vi "Main.vi"() -> ()   [LabVIEW 2021]
uses:
  Program Files (x86)/National Instruments/LabVIEW 2021/examples/Design Patterns/Queued Message Handler/support/QMH Fundamentals - Message Cluster.ctl
  <vilib>/Utility/file.llb/Write Delimited Spreadsheet (string).vi
  <vilib>/Utility/xml.llb/Write to XML File(string).vi
  <vilib>/Utility/error.llb/Error Cluster From Error Code.vi
  <vilib>/Utility/xml.llb/Read From XML File(array).vi
  <vilib>/ErrorRing/Error Ring.xnode
panel:
  in  "bt_Manuel":bool caption="Manuel"
  out "boolEmergancyStop":bool caption="Acil Stop"
  out "bool_1":bool
  out "boolPollutionIndicator":bool caption="Kirlilik \nGöstergesi"
  out "boolMotorProtectionSwitch":bool caption="Motor\nKoruma Şalteri"
  in  "Bits":bool[](array[boolean])=[FALSE, FALSE, FALSE, FALSE, FALSE, FALSE, FALSE, FALSE, FALSE, FALSE, FALSE, FALSE, TRUE, FALSE, FALSE, FALSE, FALSE, TRUE, FALSE, FALSE, FALSE, FALSE, FALSE, TRUE, FALSE, FALSE, TRUE, TRUE, FALSE]
  in  "Languages":u16(ring)
  in  "Add Image":bool
  in  "bt_reportExcel":bool caption="Rapor"
  out "imagework":picture
  out "image testprm":picture
  in  "error in":errorcluster
  in  "bt_compare":bool caption="Karşılaştır"
  in  "bt_alarms":bool caption="Alarmlar"
  in  "bt_calibration":bool caption="Kalibrasyon"
  in  "bt_testStart":bool caption="Test Başlat"
  in  "bt_testStop":bool caption="Test Bitir"
  in  "bt_testPause":bool caption="Test Durdur"
  in  "bt_testCall":bool caption="Test Çağır"
  in  "bt_stopHydraulicSystem":bool caption="Sistem Durdur"
  in  "bt_startHydraulicSystem":bool caption="Sistem Başlat"
  in  "bt_exit":bool caption="ÇIKIŞ"
  in  "bt_home":bool caption="Home Button"
  in  "Pozisyon (Position)":dbl caption="Pozisyon" format="%#_g mm"
  in  "Kuvvet (Force)":dbl caption="Kuvvet" format="%#_6g N"
  out "Display Message":string="Test Edit" caption="DURUM BİLGİSİ"
  in  "General Tab":T1(tab)=enum."KalıpSeçimi"
  in  "General Pages Tab":T1(tab)=enum."KalıpSeçimi"
  in  "bt_continue":bool
  in  "Color Box":u32(colorbox)=12441574
  in  "Test Button General":enum32{"0", "1", "2"}(tab)=enum."1"
  in  "Test Pages Tab":enum32{"0", "1", "2", "3", "4", "5"}(tab)
  in  "KALIP BİLGİLERİ":T2={"Parça No"="Deneme2", "Seri No"="1", "Müşteri"="Mercedes-Benz", "Kalıp No"="6666", "Kuvvet Limiti [kN]"="1000", "Pres Tur"="15"} caption="t"
  in  "KONTROL PARAM":T3={"Kuvvet Limit"="Deneme2", "Grafik Limit"="1"}
  in  "String 2":string caption="Hız"
  in  "String":string caption="Pozisyon"
  in  "HAREKET PROFİLİ":T4 {"Bekleme Süresi" format="%#_g s"; "S3" format="%#_g mm/s"; "BDC" format="%#_g mm"; "S2" format="%#_g mm/s"; "P1" format="%#_g mm"; "S1" format="%#_g mm/s"; "TDC" format="%#_g mm"}
  in  "Image":i32(listbox) caption="Resim Seç"
  out "2D Picture":picture
  in  "bt_controlParameters":bool caption="Kontrol Parametreleri"
  in  "bt_moldInformation":bool caption="Kalıp Bilgileri"
  in  "bt_motionProfile":bool caption="Hareket Profili"
  in  "bt_recipeSave":bool caption="Kaydet"
  in  "bt_recipeSend":bool caption="Çalışmaya Gönder"
  in  "bt_recipeDelete":bool caption="Sil"
  in  "bt_graphLimited":bool caption="Grafik Sınırlayıcı"
  in  "bt_imageUpload":bool caption="Resim Yükle"
  in  "bt_newRecipe":bool caption="Yeni Kayıt"
  in  "Test Button Tab":enum32{"0", "1", "2", "3", "4", "5"}(tab)=enum."3"
  in  "bt_registrationPage":bool caption="Kayıt Sayfası"
  in  "bt_moldRecipeSearch":bool caption="Kalıp Ara"
  in  "searchRecipe":string="Deneme3"
  in  "moldSelection":i32(listbox)=2 caption="KALIP SEÇİMİ"
  in  "Mold Choice Tab":enum32{"0", "1"}(tab)=enum."1"
  out "pieceNo":string="Deneme2" caption="Parça No"
  out "serialNo":string="1" caption="Seri No"
  in  "bt_testEdit":bool caption="Testi Düzenle"
  out "Display Message 2":string="Test Edit" caption="Son Alarm"
  out "XY Graph":cluster{"X":dbl, "Y":dbl}[](graph)
  out "KALIP BİLGİLERİ-ÇALIŞMAs":T2={"Parça No"="Deneme2", "Seri No"="1", "Müşteri"="Mercedes-Benz", "Kalıp No"="6666", "Kuvvet Limiti [kN]"="1000", "Pres Tur"="15"} caption="KALIP BİLGİLERİ"
  in  "poliTestCheckbox":bool caption="Çoklu Test"
  in  "TEST PARAMETRELERİ":T5 caption="t" {"adet" format="%#_g mm"; "Min Kuvvet" format="%#_g kN"; "Max Kuvvet" format="%#_g kN"; "Min Pozisyon" format="%#_g mm"; "Max Pozisyon" format="%#_g mm"; "Kuvvet" format="%#_g kN"; "anlıkKuvvet" format="%#_g s"; "Hız" format="%#_g mm/s"; "tur" format="%#_g mm"}
  out "Comparexy":T6(graph)
  in  "deleteReferance":bool caption="Sil"
  out "Grafik Sayısı":string="2"
  in  "graphicReset":bool caption="Grafik Reset"
  in  "addReferance":bool caption="Grafik Ekle"
  in  "Alt Limit":string="30"
  in  "Referans Veriler":i32(listbox)=1
  in  "bt_AlarmsRemove":bool caption="REMOVE"
  in  "Alarms":i32(listbox) caption="ALARMLAR"
  in  "bt_CalibrationManuel":bool caption="MANUEL"
  in  "bt_CalibrationSave":bool caption="KAYDET"
  out "Cluster 3":T7 {"park_Position" format="%#_g s"; "decomp_CycleTime" format="%#_g s"; "YEDEK" format="%#_g s"; "YEDEK" format="%#_g s"; "YEDEK" format="%#_g h"; "decomp_Cycle" format="%#_g s"; "p6_Druck" format="%#_g s"; "auffahren_Druck" format="%#_g h"; "press_Druck" format="%#_g s"; "langsam_Druck" format="%#_g mm"; "Schnellabdruck" format="%#_g bar"; "low_Temp" format="%#_g kN"; "fan_StopTemp" format="%#_g bar"; "fan_StartTemp" format="%#_g mm"}
  in  "Cluster 2":T8
  out "Cluster":T9 {"YEDEK" format="%#_g s"; "YEDEK" format="%#_g bar"; "YEDEK" format="%#_g kN"; "Wait" format="%#_g s"; "working_Time" format="%#_g h"; "Time" format="%#_g s"; "min_PosD" format="%#_g mm"; "pressure_Bd" format="%#_g bar"; "Kraftd" format="%#_g kN"; "pressure_Name" format="%#_g bar"; "Position" format="%#_g mm"}
  out "Table Control 2":string[][](table) caption="Table Control"
  out "Table Control":string[][](table)
  # "NOTLAR\n1- Otomatik sayfası eklenecek (climatic testteki gibi)\n2- Ayarlar sayfasındaki fan start clusteri gizle ve Pega climaticteki kalibrasyon sayfasındaki\ngibi input ve output boolean değişkenleri ekle\n3- Grafik sınırlayıcıyı fıratın anlattığı ve attığı videolardaki gibi yap\n4-"
  # "V 0.0.0.1"
  # "MSP-120-S-HCD\n120kN Servo Press"
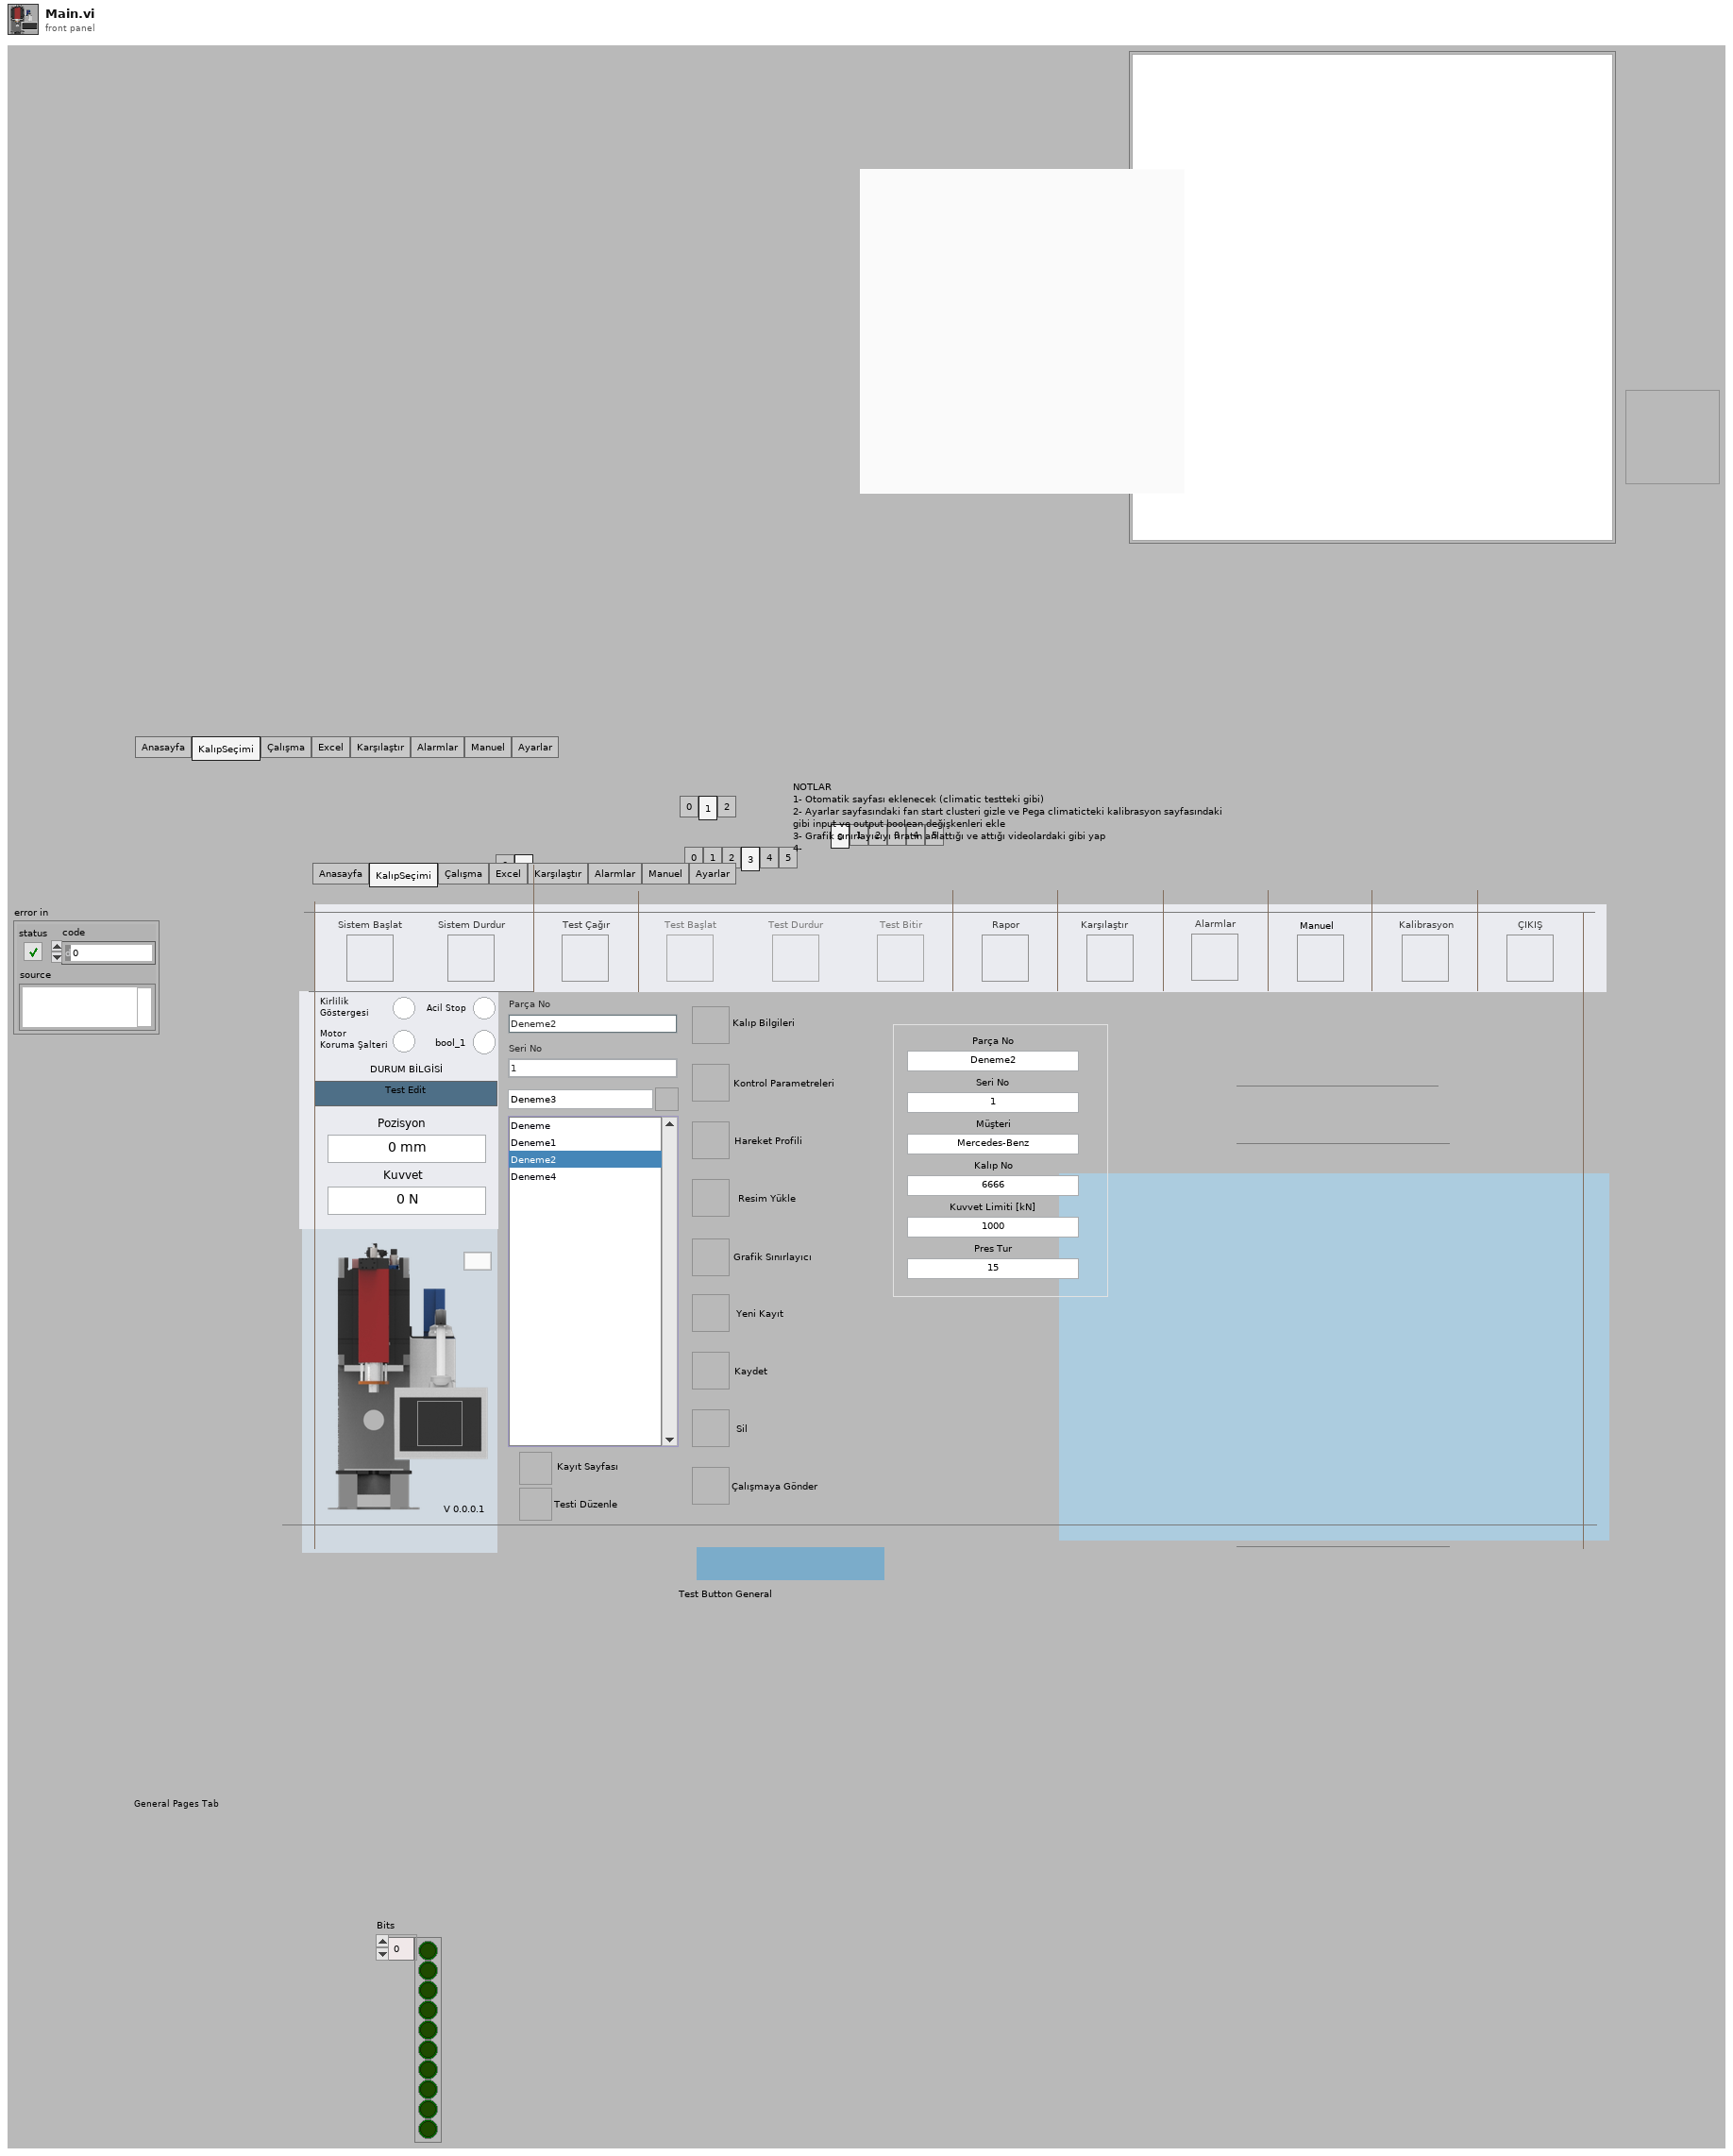
[diagram p1: front panel]
types:
  T1 = enum32{"Anasayfa", "KalıpSeçimi", "Çalışma", "Excel", "Karşılaştır", "Alarmlar", "Manuel", "Ayarlar"}
  T2 = cluster{"Parça No":string, "Seri No":string, "Müşteri":string, "Kalıp No":string, "Kuvvet Limiti [kN]":string, "Pres Tur":string}
  T3 = cluster{"Kuvvet Limit":string, "Grafik Limit":string}
  T4 = cluster{"TDC":dbl, "S1":dbl, "P1":dbl, "S2":dbl, "BDC":dbl, "S3":dbl, "Bekleme Süresi":dbl}
  T5 = cluster{"tur":dbl, "Hız":dbl, "anlıkKuvvet":dbl, "Kuvvet":dbl, "Max Pozisyon":dbl, "Min Pozisyon":dbl, "Max Kuvvet":dbl, "Min Kuvvet":dbl, "adet":dbl}
  T6 = cluster{"Item Names":dbl[], "Item Names":dbl[]}[]
  T7 = cluster{"fan_StartTemp":dbl, "fan_StopTemp":dbl, "over_Temp":dbl, "low_Temp":dbl, "Schnellabdruck":dbl, "langsam_Druck":dbl, "press_Druck":dbl, "auffahren_Druck":dbl, "p5_Druck":dbl, "p6_Druck":dbl, "decomp_Cycle":dbl, "YEDEK":dbl, "YEDEK":dbl, "YEDEK":dbl, "YEDEK":dbl, "decomp_CycleTime":dbl, "park_Position":dbl}
  T8 = cluster{"jog_Press":bool, "Fgrenze":bool, "start_HoldTime":bool, "move_DoneForce":bool, "hold_TimeDone":bool, "start_Decomp":bool, "decompJog":bool, "Startup":bool, "Motion":bool, "Lamp":bool, "reset_Axis":bool, "YEDEK":bool, "YEDEK":bool, "YEDEK":bool}
  T9 = cluster{"Position":dbl, "pressure_Name":dbl, "total_Parts":dbl, "Kraftd":dbl, "pressure_Bd":dbl, "min_PosD":dbl, "Time":dbl, "working_Time":dbl, "max_Force":dbl, "Wait":dbl, "YEDEK":dbl, "YEDEK":dbl, "YEDEK":dbl, "YEDEK":dbl}
  T10 = typedef "QMH Fundamentals - Message Cluster.ctl" = cluster{"Message":string, "Message Data":variant}
  T11 = enum16{"open", "replace", "create", "open or create", "replace or create", "replace or create with confirmation"}
  T12 = cluster{"Parça No":string, "Seri No":string, "Müşteri":string, "Kalıp No":string, "Kuvvet Limiti [kN]":string, "Kuvvet Limiti [kN] 2":string}
  T13 = cluster{"KALIP BİLGİLERİ 2":cluster{"Parça No":string, "Seri No":string, "Müşteri":string, "Kalıp No":string, "Kuvvet Limiti [kN]":string, "Kuvvet Limiti [kN] 2":string}, "Parça No":string, "Seri No":string, "KALIP BİLGİLERİ":cluster{"Kuvvet Limiti [kN]":string, "Kuvvet Limiti [kN] 2":string}, "HAREKET PROFİLİ":cluster{"TDC":dbl, "S1":dbl, "P1":dbl, "S2":dbl, "BDC":dbl, "S3":dbl, "Bekleme Süresi":dbl}, "new picture":picture, "picture index":dbl}
  T14 = cluster{"Kuvvet Limiti [kN]":string, "Kuvvet Limiti [kN] 2":string}
  T15 = enum8{"Enabled", "Disabled", "Disabled and Grayed Out"}
  T16 = typedef "imagedata.ctl" = cluster{"image type":i32, "image depth":i32, "image":u8[], "mask":u8[], "colors":u32[], "Rectangle":cluster{"left":i16, "top":i16, "right":i16, "bottom":i16}}
  T17 = cluster{"Parça No":string, "Seri No":string, "Müşteri":string, "Kalıp No":string, "Kuvvet Limiti [kN]":string}
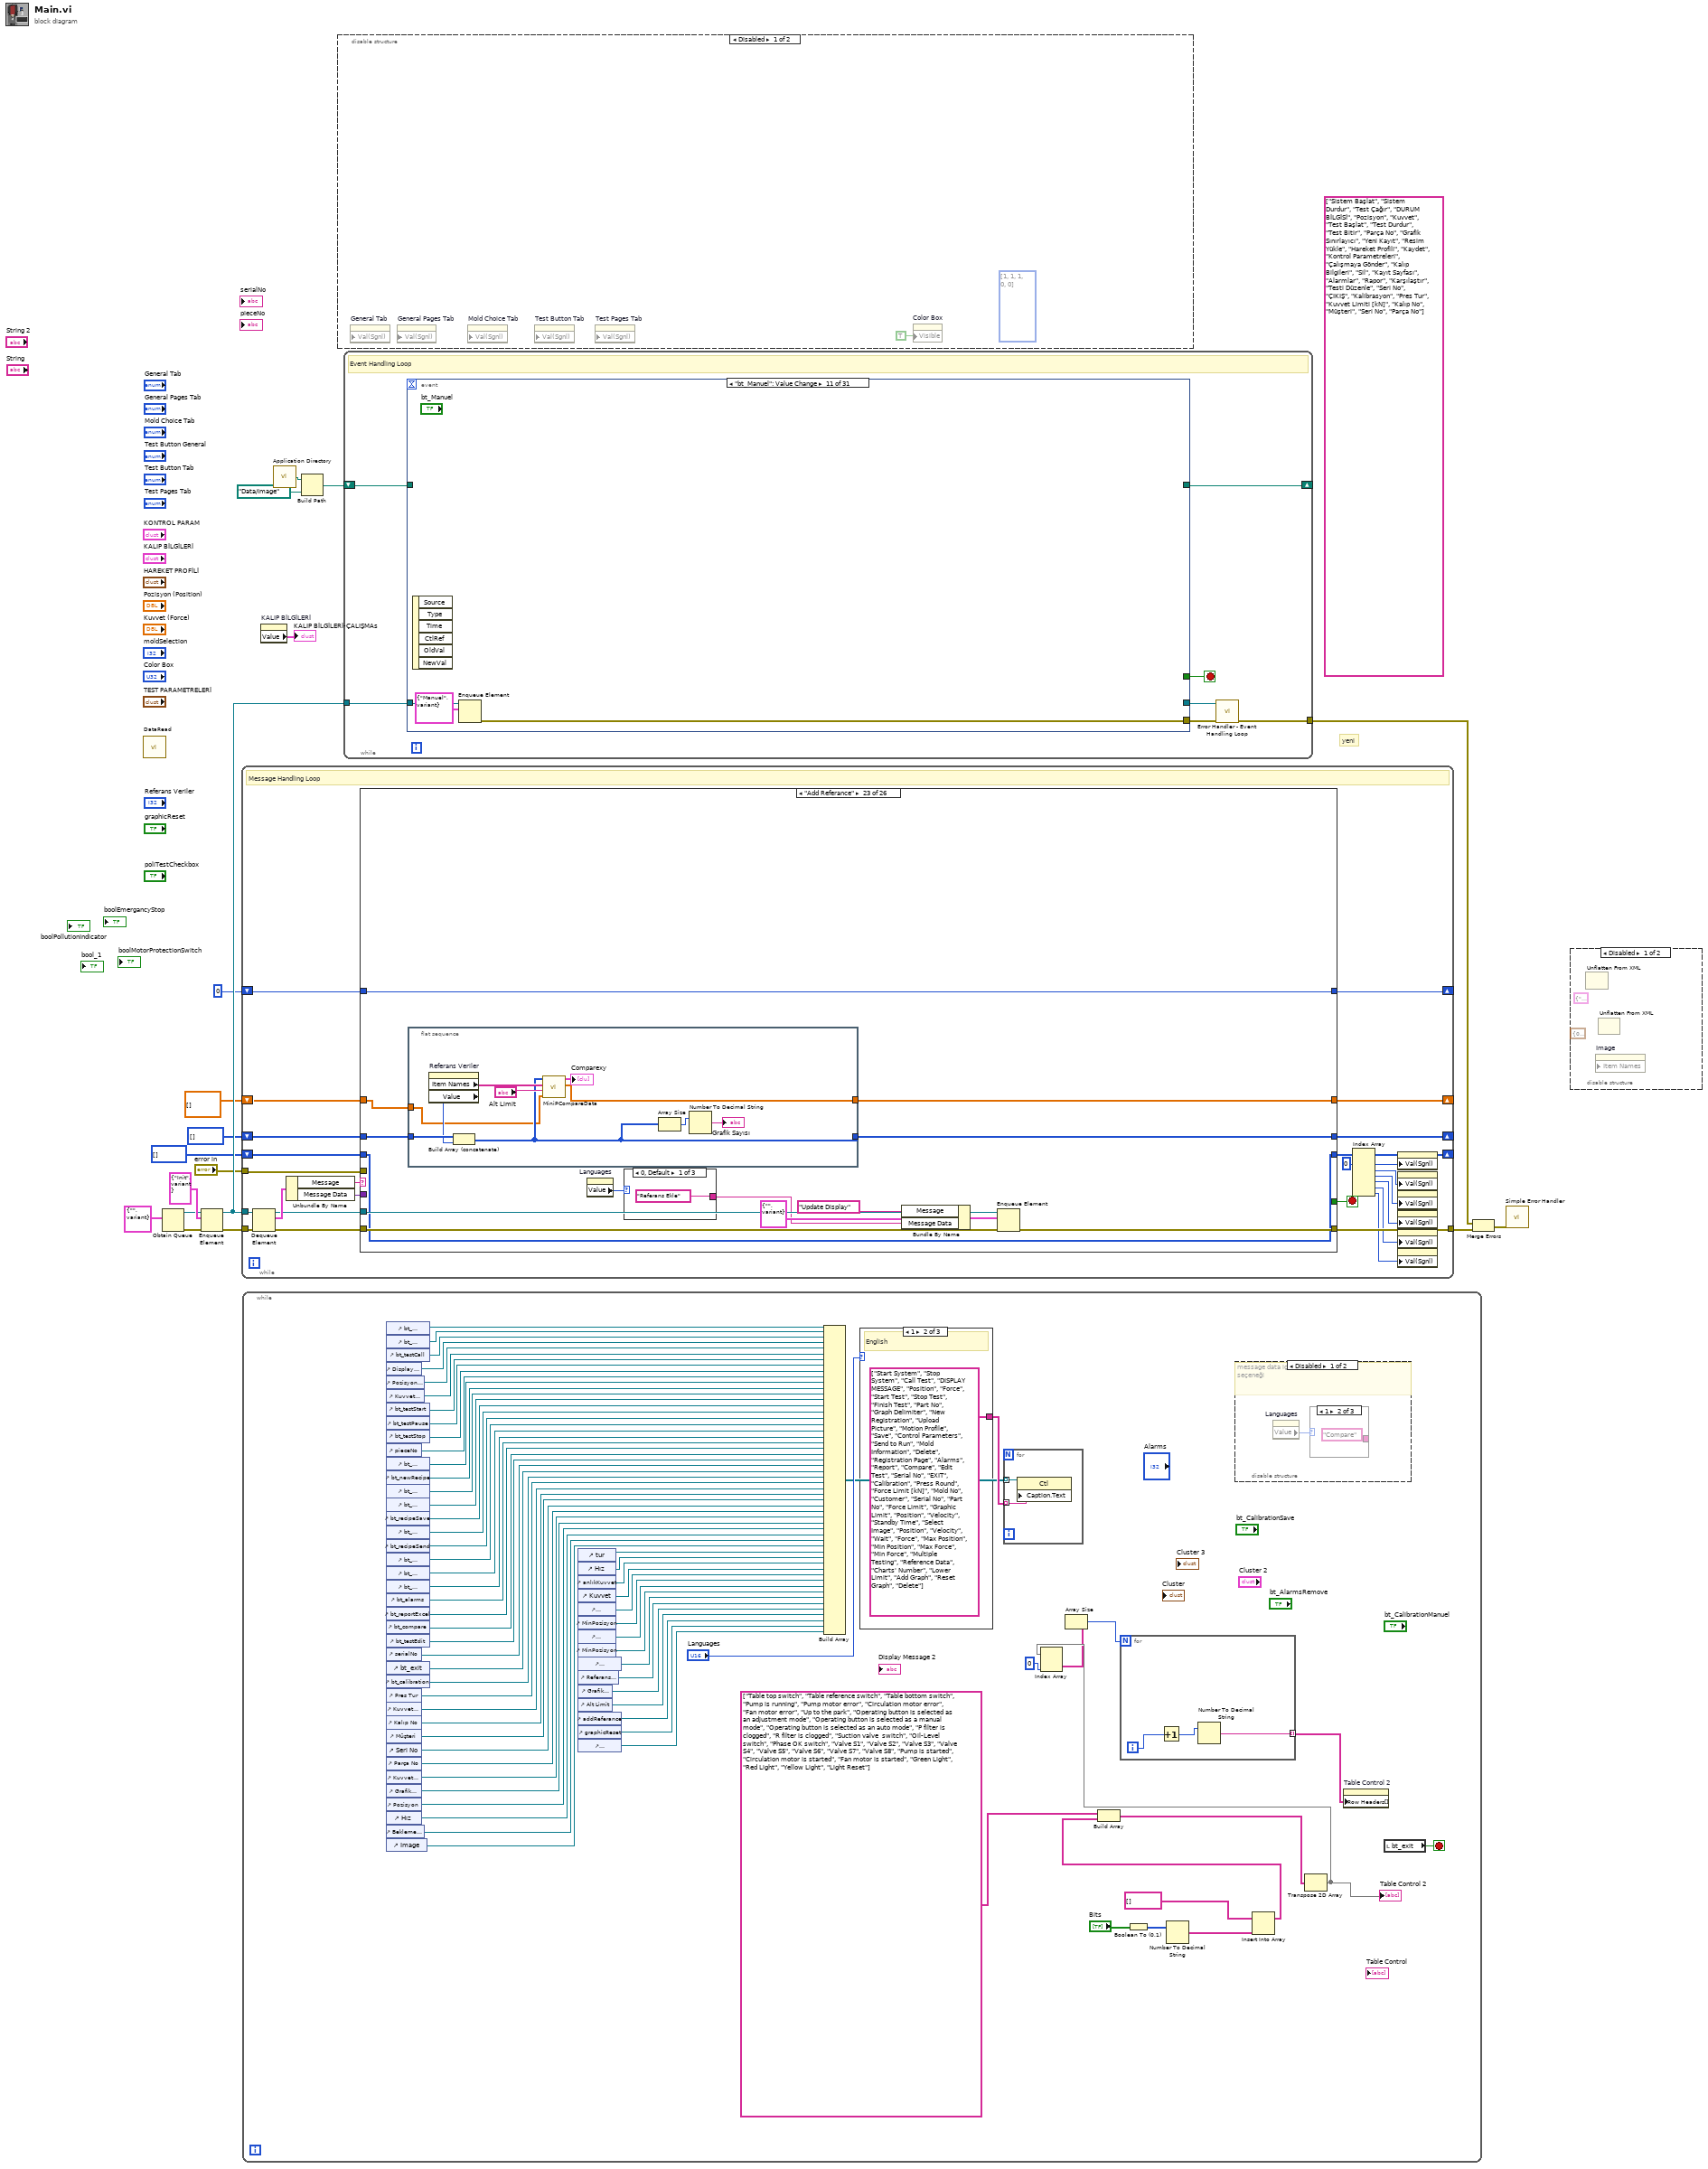
[diagram p0: block diagram]
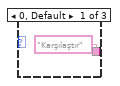
[diagram p2: hidden frame]
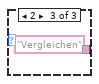
[diagram p3: hidden frame]
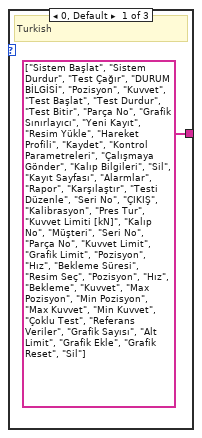
[diagram p5: hidden frame]
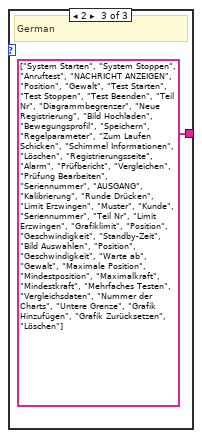
[diagram p6: hidden frame]
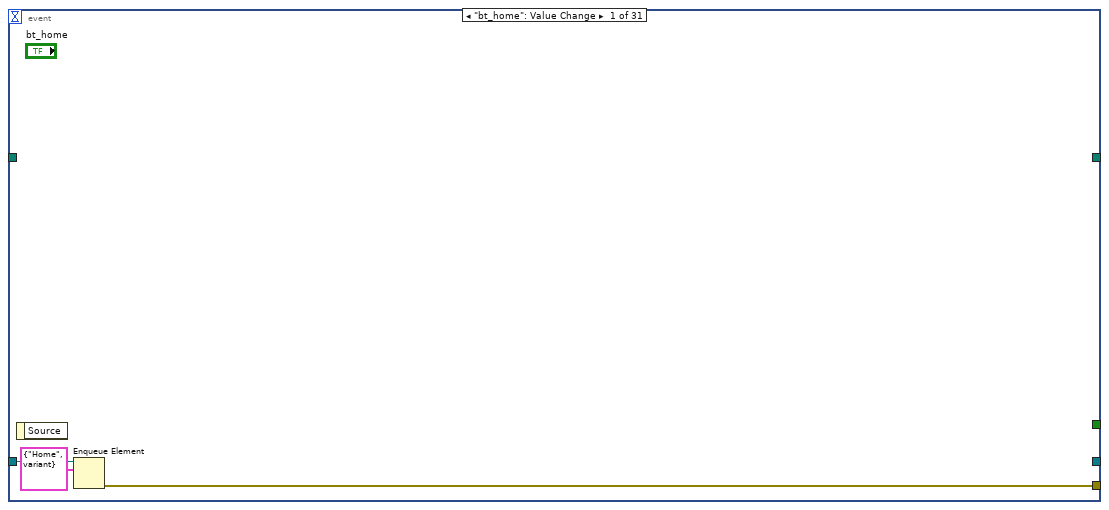
[diagram p9: hidden frame]
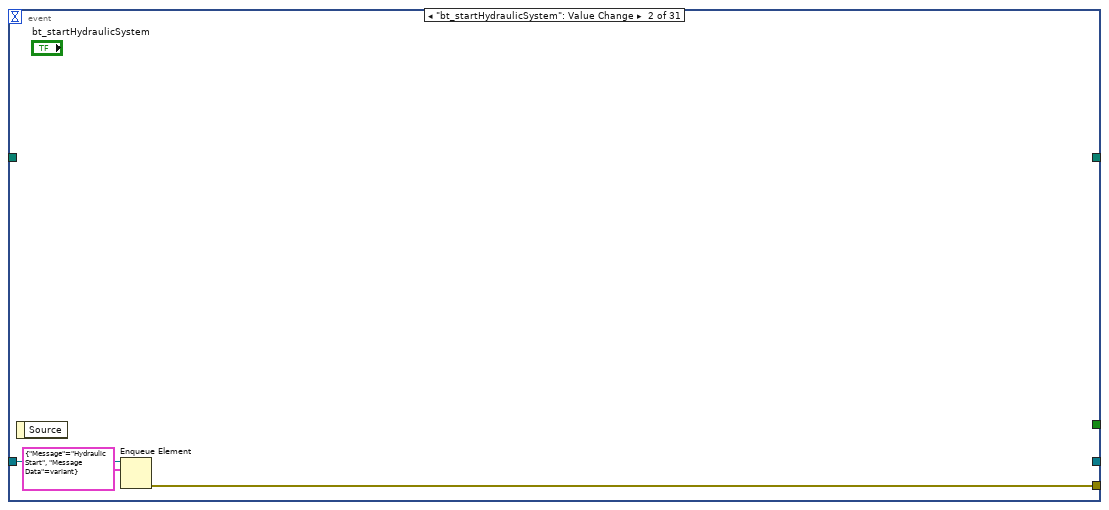
[diagram p10: hidden frame]
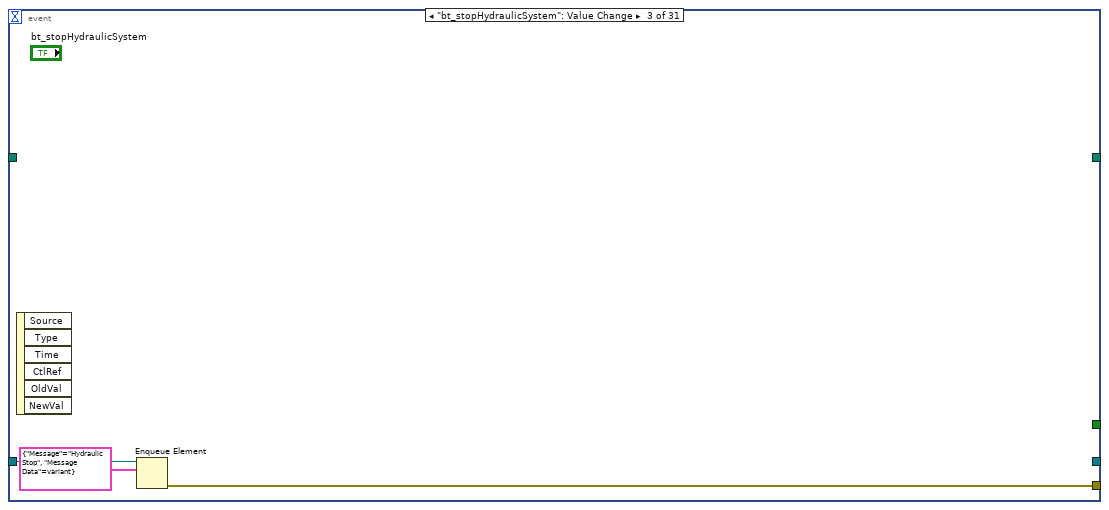
[diagram p11: hidden frame]
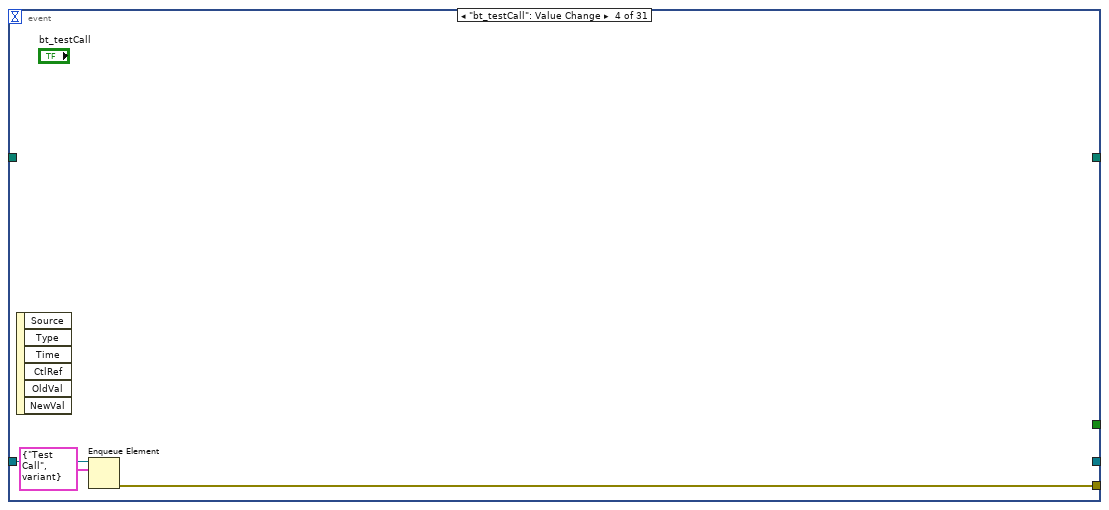
[diagram p12: hidden frame]
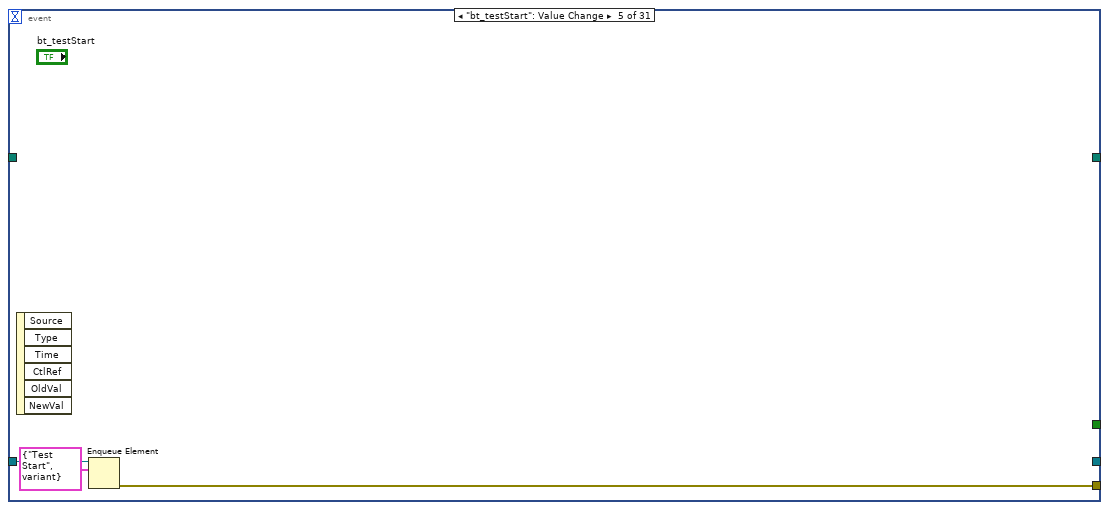
[diagram p13: hidden frame]
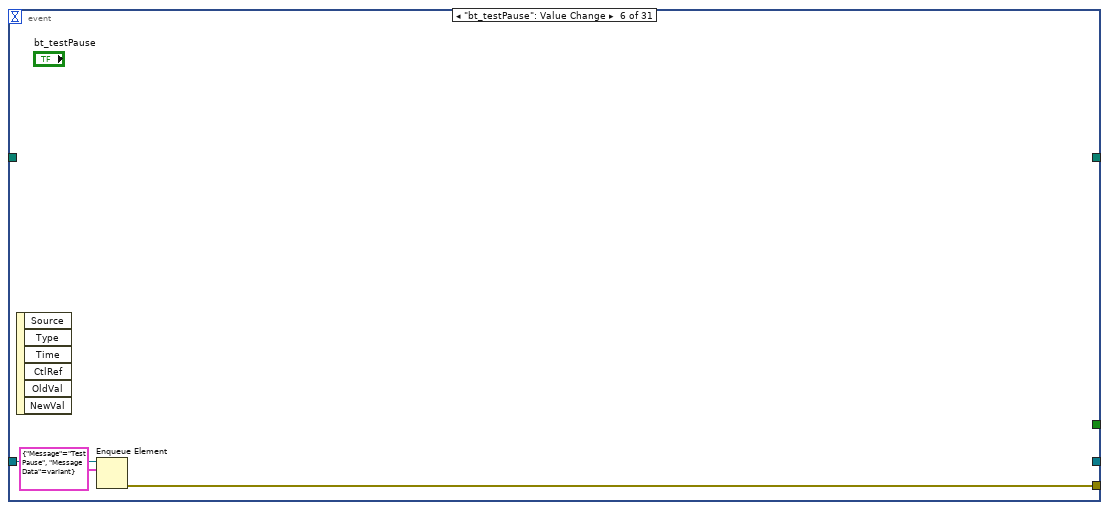
[diagram p14: hidden frame]
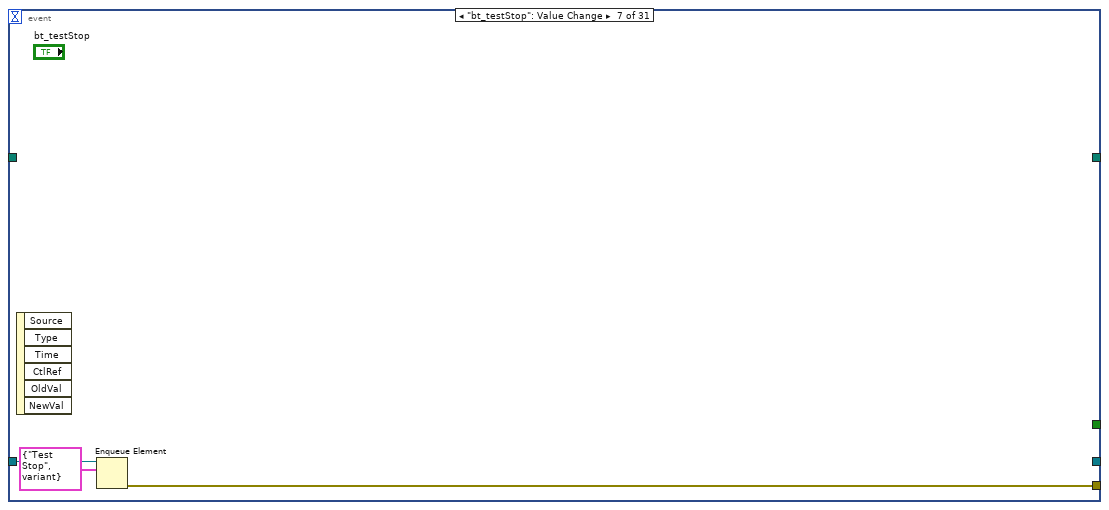
[diagram p15: hidden frame]
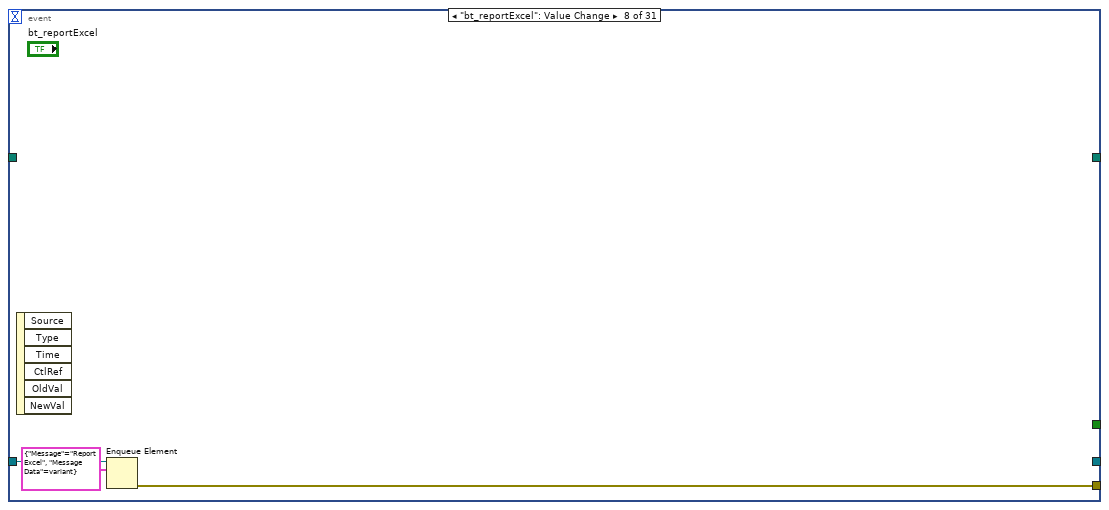
[diagram p16: hidden frame]
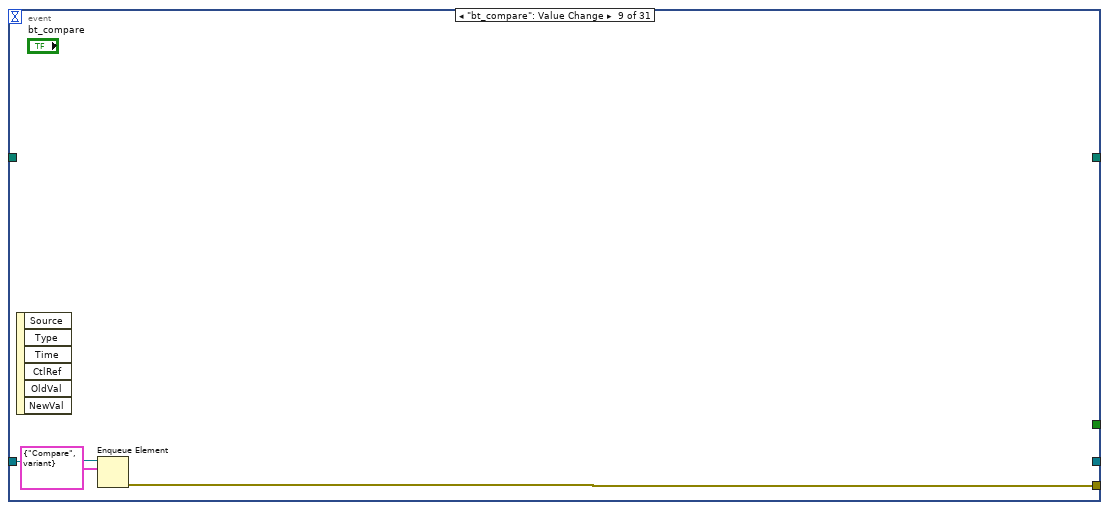
[diagram p17: hidden frame]
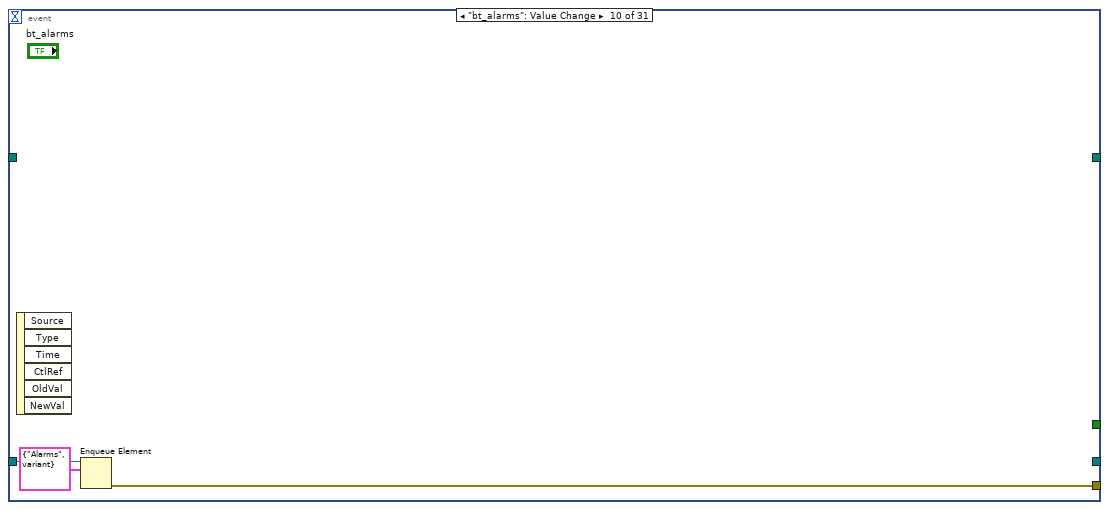
[diagram p18: hidden frame]
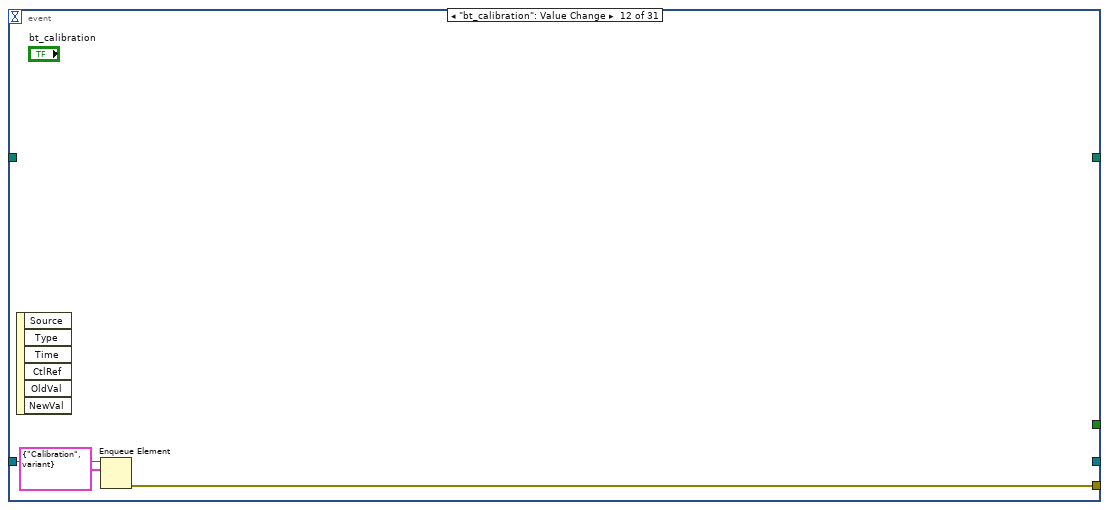
[diagram p19: hidden frame]
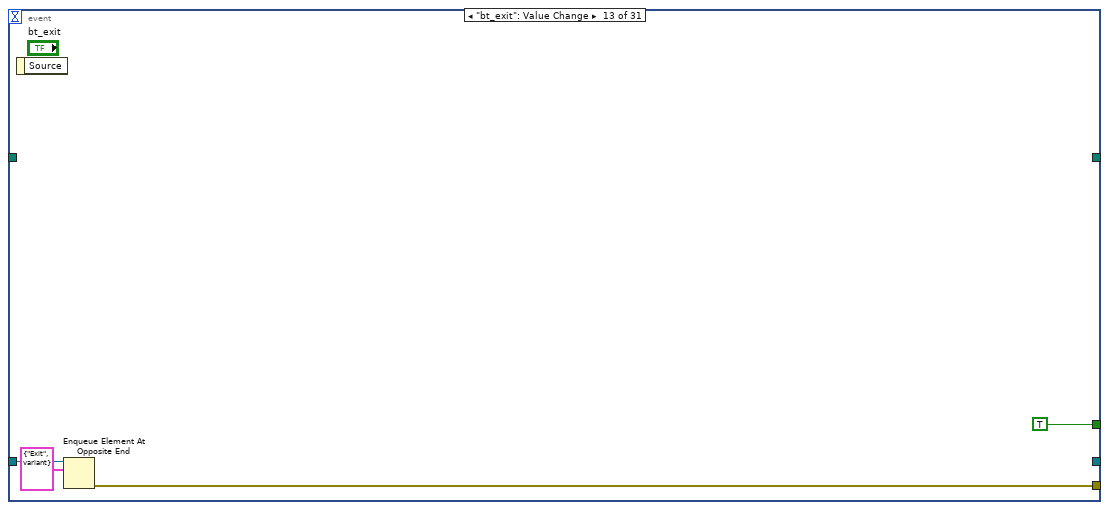
[diagram p20: hidden frame]
diagram:
  (unwired) string[] ["Sistem Başlat", "Sistem Durdur", "Test Çağır", "DURUM BİLGİSİ", "Pozisyon", "Kuvvet", "Test Başlat", "Test Durdur", "Test Bitir", "Parça No", "Grafik Sınırlayıcı", "Yeni Kayıt", "Resim Yükle", "Hareket Profili", "Kaydet", "Kontrol Parametreleri", "Çalışmaya Gönder", "Kalıp Bilgileri", "Sil", "Kayıt Sayfası", "Alarmlar", "Rapor", "Karşılaştır", "Testi Düzenle", "Seri No", "ÇIKIŞ", "Kalibrasyon", "Pres Tur", "Kuvvet Limiti [kN]", "Kalıp No", "Müşteri", "Seri No", "Parça No"] ("appended array")
  # "yeni"
  n1 = call "DataRead.vi"() -> ()  [unwired: 12 in]
  n2 = Obtain Queue(element data type=T10 {"Message"="", "Message Data"=variant} ("Message Cluster")) -> (queue out=w11:refnum<queue>, error out=w10:errorcluster)  [unwired: 4 in, 1 out]
  n3 = Enqueue Element(queue=w11, element=T10 {"Message"="Init", "Message Data"=variant}, error in (no error)=w10) -> (queue out=w15:refnum<queue>, error out=w16:errorcluster)  [unwired: 1 in, 1 out]
  n4 = while {
    tunnel: w15 -> [w40]
    tunnel: w16 -> [w41]
    tunnel: [w42] -> w18
    tunnel: "error in" -> [w34]
    shift-right: [w31] -> _
    shift-left: i32[] [] -> [w30]
    shift-right: [w23] -> _
    shift-left: i32[] [] -> [w24]
    shift-right: [w22] -> _
    shift-left: dbl[][] [] ("output array 3") -> [w19]
    shift-right: [w20] -> _
    shift-left: 0 -> [w21]
    stop <- w43 stop-if-true
    # "Message Handling Loop"
    n5 = Dequeue Element(queue=w40, error in (no error)=w41) -> (queue out=w38:refnum<queue>, element=w39:T10, error out=w37:errorcluster)  [unwired: 1 in, 1 out]
    n6 = Unbundle By Name(w39) -> ("Message"=w36:string, "Message Data"=w35:variant)
    n7 = case "Message Cases" shown="\"Add Referance\"" w36 {
      selector: w36 -> [_ _ _ _ _ _ _ _ _ _ _ _ _ _ _ _ _ _ _ _ _ _ _ _ _ w671]
      tunnel: w38 -> [_ w63 w78 w93 w113 w128 w143 w158 w214 w252 w290 w306 w321 w334 w349 w366 w418 w433 w456 w505 w558 w601 w618 w645 _ _]
      tunnel: w37 -> [w51 w61 w76 w91 w111 w126 w141 w156 w212 w250 w288 w304 w319 w331 w347 w364 w416 w431 w455 w504 w556 w599 w616 w643 w664 w670]
      tunnel: [w51 w62 w77 w92 w112 w127 w142 w157 w213 w251 w289 w305 w320 w332 w348 w365 w417 w432 w442 w492 w557 w600 w617 w644 w662 w670] -> w42
      tunnel: [_ _ _ _ _ _ _ _ _ _ _ _ _ TRUE _ _ _ _ _ _ _ _ _ _ _ _] -> w43
      tunnel: w35 -> [_ _ _ _ _ _ _ _ _ _ _ _ _ _ _ _ _ _ _ _ _ _ _ _ w663 _]
      tunnel: w34 -> [_ _ _ _ _ _ _ _ w163 _ w279 w295 _ _ _ _ _ _ w451 _ _ _ _ _ _ _]
      tunnel: [i32[] [0, 0, 0, 0, 0] i32[] [0, 0, 0, 0, 0] w72 w87 w103 w122 w137 w152 w208 i32[] [4, 4, 0, 1, 0] i32[] [5, 5, 0, 1, 0] i32[] [6, 6, 0, 1, 0] i32[] [7, 7, 0, 1, 0] w330 i32[] [1, 1, 0, 5, 5] w357 w407 i32[] [1, 1, 1, 1, 0, 0] w446 w483 w552 i32[] [2, 2, 1, 1, 0] w612 w639 w660 w668] -> w31
      tunnel: w30 -> [_ _ w72 w87 w102 w122 w137 w152 w208 _ _ _ _ w330 _ w358 w412 _ w445 w488 w552 _ w612 w639 w660 w668]
      tunnel: w24 -> [w48 w56 w71 w86 w101 w121 w136 w151 w207 w245 w283 w299 w314 w329 w342 w359 w406 w426 w441 w482 w551 w594 w611 w638 w659 w667]
      tunnel: [w48 w56 w71 w86 w101 w121 w136 w151 w207 w245 w283 w299 w314 w329 w342 w359 w406 w426 w441 w482 w551 w594 w610 w636 w659 w667] -> w23
      tunnel: w19 -> [w45 w55 w70 w85 w100 w120 w135 w150 w175 w244 w282 w298 w313 w328 w341 w356 w405 w425 w440 w481 w550 w593 w605 w635 w657 w666]
      tunnel: [w45 w55 w70 w85 w100 w120 w135 w150 w175 w244 w282 w298 w313 w328 w341 w356 w405 w425 w440 w481 w550 w593 w606 w634 w657 w666] -> w22
      tunnel: w21 -> [w44 w54 w69 w84 w99 w119 w134 w149 w169 w243 w281 w297 w312 w327 w340 w355 w404 w424 w439 w480 w549 w592 w609 w637 w656 w665]
      tunnel: [w44 w54 w69 w84 w99 w119 w134 w149 w165 w243 w281 w297 w312 w327 w340 w355 w404 w424 w439 w480 w549 w592 w609 w637 w656 w665] -> w20
      frame "Init" {
        # "Initialize - Perform any initialization code for your application here. In this example, the only initialization required is setting the Display Message indicator value to an empty string."
        n8 = property on="moldSelection" class="LstBox (strict)"("Value"=nan) -> ()  [unwired: 2 in, 2 out]
        n9 = property on="Test Button General" class="TabCtl (strict)"("Val(Sgnl)"=enum32{"0", "1", "2"}."0" ("Value (Signaling)")) -> ()  [unwired: 2 in, 2 out]
        n10 = local write "Display Message"("") -> ()
      }
      frame "Home" {
        # "Action 1 - Send an \"Update Display\" message indicating which button was pressed. Note that a string is sent as the Message Data along with the \"Update Display\" message."
        n11 = property on="Languages" class="Ring (strict)"() -> ("Value"=w53:u16)  [unwired: 2 in, 2 out]
        n12 = case shown="0, Default" w53 {
          tunnel: ["Ev" ("L10n_Action 2 Pressed") "Home" ("L10n_Action 2 Pressed") "Heim" ("L10n_Action 2 Pressed")] -> w52
          frame 0, Default {
          }
          frame 1 {
          }
          frame 2 {
          }
        }
        n13 = Bundle By Name(cluster=T10 {"Message"="", "Message Data"=variant} ("Message Cluster"), "Message"="Update Display", "Message Data"=w52) -> (w58:T10)
        n14 = Enqueue Element(queue=w63, element=w58, error in (no error)=w61) -> (error out=w62:errorcluster)  [unwired: 1 in, 2 out]
      }
      frame "Hydraulic Start" {
        # "Action 1 - Send an \"Update Display\" message indicating which button was pressed. Note that a string is sent as the Message Data along with the \"Update Display\" message."
        n15 = property on="Languages" class="Ring (strict)"() -> ("Value"=w68:u16)  [unwired: 2 in, 2 out]
        n16 = case shown="2" w68 {
          tunnel: ["Hidrolik Başlat" ("L10n_Action 2 Pressed") "Hydraulic Start" ("L10n_Action 2 Pressed") "Hydraulik Starten" ("L10n_Action 2 Pressed")] -> w67
          frame 0, Default {
          }
          frame 1 {
          }
          frame 2 {
          }
        }
        n17 = Bundle By Name(cluster=T10 {"Message"="", "Message Data"=variant} ("Message Cluster"), "Message"="Update Display", "Message Data"=w67) -> (w73:T10)
        n18 = Enqueue Element(queue=w78, element=w73, error in (no error)=w76) -> (error out=w77:errorcluster)  [unwired: 1 in, 2 out]
      }
      frame "Hydraulic Stop" {
        # "Action 2 - Send an \"Update Display\" message indicating which button was pressed. Note that a string is sent as the Message Data along with the \"Update Display\" message."
        n19 = property on="Languages" class="Ring (strict)"() -> ("Value"=w83:u16)  [unwired: 2 in, 2 out]
        n20 = case shown="2" w83 {
          tunnel: ["Hidrolik Durdur" ("L10n_Action 2 Pressed") "Hydraulic Stop" ("L10n_Action 2 Pressed") "Hydraulik Stoppen" ("L10n_Action 2 Pressed")] -> w82
          frame 0, Default {
          }
          frame 1 {
          }
          frame 2 {
          }
        }
        n21 = Bundle By Name(cluster=T10 {"Message"="", "Message Data"=variant} ("Message Cluster"), "Message"="Update Display", "Message Data"=w82) -> (w88:T10)
        n22 = Enqueue Element(queue=w93, element=w88, error in (no error)=w91) -> (error out=w92:errorcluster)  [unwired: 1 in, 2 out]
      }
      frame "Test Call" {
        # "Action 2 - Send an \"Update Display\" message indicating which button was pressed. Note that a string is sent as the Message Data along with the \"Update Display\" message."
        n23 = property on="Languages" class="Ring (strict)"() -> ("Value"=w98:u16)  [unwired: 2 in, 2 out]
        n24 = case shown="2" w98 {
          tunnel: ["Test Çağır" ("L10n_Action 2 Pressed") "Call Test" ("L10n_Action 2 Pressed") "Anruftest" ("L10n_Action 2 Pressed")] -> w97
          frame 0, Default {
          }
          frame 1 {
          }
          frame 2 {
          }
        }
        n25 = Replace Array Subset(array=w102, new element #1=1 ("new element/subarray"), index #1=0 ("index"), new element #2=1 ("new element/subarray"), index #2=1 ("index")) -> (w103:i32[])
        n26 = Bundle By Name(cluster=T10 {"Message"="", "Message Data"=variant} ("Message Cluster"), "Message"="Update Display", "Message Data"=w97) -> (w108:T10)
        n27 = Enqueue Element(queue=w113, element=w108, error in (no error)=w111) -> (error out=w112:errorcluster)  [unwired: 1 in, 2 out]
      }
      frame "Test Start" {
        # "Action 2 - Send an \"Update Display\" message indicating which button was pressed. Note that a string is sent as the Message Data along with the \"Update Display\" message."
        n28 = property on="Languages" class="Ring (strict)"() -> ("Value"=w118:u16)  [unwired: 2 in, 2 out]
        n29 = case shown="2" w118 {
          tunnel: ["Test Başlat" ("L10n_Action 2 Pressed") "Test Start" ("L10n_Action 2 Pressed") "Test Starten" ("L10n_Action 2 Pressed")] -> w117
          frame 0, Default {
          }
          frame 1 {
          }
          frame 2 {
          }
        }
        n30 = Bundle By Name(cluster=T10 {"Message"="", "Message Data"=variant} ("Message Cluster"), "Message"="Update Display", "Message Data"=w117) -> (w123:T10)
        n31 = Enqueue Element(queue=w128, element=w123, error in (no error)=w126) -> (error out=w127:errorcluster)  [unwired: 1 in, 2 out]
      }
      frame "Test Pause" {
        # "Action 2 - Send an \"Update Display\" message indicating which button was pressed. Note that a string is sent as the Message Data along with the \"Update Display\" message."
        n32 = property on="Languages" class="Ring (strict)"() -> ("Value"=w133:u16)  [unwired: 2 in, 2 out]
        n33 = case shown="0, Default" w133 {
          tunnel: ["Test Durdur" ("L10n_Action 2 Pressed") "Test Pause" ("L10n_Action 2 Pressed") "Test Stoppen" ("L10n_Action 2 Pressed")] -> w132
          frame 0, Default {
          }
          frame 1 {
          }
          frame 2 {
          }
        }
        n34 = Bundle By Name(cluster=T10 {"Message"="", "Message Data"=variant} ("Message Cluster"), "Message"="Update Display", "Message Data"=w132) -> (w138:T10)
        n35 = Enqueue Element(queue=w143, element=w138, error in (no error)=w141) -> (error out=w142:errorcluster)  [unwired: 1 in, 2 out]
      }
      frame "Test Stop" {
        # "Action 2 - Send an \"Update Display\" message indicating which button was pressed. Note that a string is sent as the Message Data along with the \"Update Display\" message."
        n36 = property on="Languages" class="Ring (strict)"() -> ("Value"=w148:u16)  [unwired: 2 in, 2 out]
        n37 = case shown="2" w148 {
          tunnel: ["Test Bitir" ("L10n_Action 2 Pressed") "Test Beenden" ("L10n_Action 2 Pressed") "Finish Test" ("L10n_Action 2 Pressed")] -> w147
          frame 0, Default {
          }
          frame 1 {
          }
          frame 2 {
          }
        }
        n38 = Bundle By Name(cluster=T10 {"Message"="", "Message Data"=variant} ("Message Cluster"), "Message"="Update Display", "Message Data"=w147) -> (w153:T10)
        n39 = Enqueue Element(queue=w158, element=w153, error in (no error)=w156) -> (error out=w157:errorcluster)  [unwired: 1 in, 2 out]
      }
      frame "Report Excel" {
        # "Action 2 - Send an \"Update Display\" message indicating which button was pressed. Note that a string is sent as the Message Data along with the \"Update Display\" message."
        n40 = property on="Languages" class="Ring (strict)"(error in=w163) -> ("Value"=w164:u16)  [unwired: 1 in, 2 out]
        n41 = Increment(x=w169) -> (x+1=w165:i32)
        n42 = case shown="2" w164 {
          tunnel: ["Excele Raporla" ("L10n_Action 2 Pressed") "Report Excel" ("L10n_Action 2 Pressed") "Prüfbericht Excel" ("L10n_Action 2 Pressed")] -> w162
          frame 0, Default {
          }
          frame 1 {
          }
          frame 2 {
          }
        }
        n43 = Number To Decimal String(number=w165) -> (decimal integer string=w167:string)  [unwired: 1 in]
        n44 = Bundle By Name(cluster=T10 {"Message"="", "Message Data"=variant} ("Message Cluster"), "Message"="Update Display", "Message Data"=w162) -> (w209:T10)
        n45 = disable-structure shown="Disabled" {
          frame Disabled {
            (unwired) dbl[][] [[244.257944, 45.058472], [244.257944, 45.058472], [244.507425, 58.662598], [244.757021, 77.658325], [245.006311, 94.001465], [245.25667, 114.316162], [245.507105, 131.029785], [245.757044, 151.04895], [246.006906, 167.49231], [246.256769, 187.022217], [246.507318, 202.838623], [246.757372, 221.95752], [247.006471, 237.069092], [247.257021, 255.672485], [247.507189, 270.313477], [247.757128, 288.54126], [248.007219, 302.773437], [248.2567, 320.695068], [248.507364, 334.658569], [248.757532, 352.358887], [249.00667, 366.036377], [249.257448, 383.486328], [249.507044, 397.035278], [249.757326, 414.338745], [250.007417, 427.50415], [250.256822, 444.507324], [250.507562, 457.680054], [250.757463, 474.576172], [251.00683, 487.561768], [251.257379, 504.411011], [251.507013, 517.157349], [251.757181, 533.88916], [252.007463, 546.530029], [252.256868, 563.121338], [252.507532, 575.629883], [252.757318, 592.188599], [253.006723, 604.656616], [253.257387, 621.057129], [253.507326, 633.444458], [253.757112, 649.878906], [254.007547, 662.192505], [254.25699, 678.359985], [254.507463, 690.679443], [254.757402, 706.931396], [255.006807, 719.049927], [255.257395, 735.057617], [255.507257, 747.286377], [255.757273, 763.268311], [256.007631, 775.393555], [256.256883, 791.341064], [256.507433, 803.436523], [256.757486, 819.349731], [257.006853, 831.404297], [257.257326, 847.233398], [257.507189, 859.23291], [257.75728, 875.164185], [258.007601, 887.022461], [258.256853, 902.898071], [258.507364, 914.703979], [258.757532, 930.603638], [259.006784, 942.289917], [259.257372, 958.166626], [259.507234, 969.790161], [259.757402, 985.563843], [260.007379, 997.39856], [260.256746, 1013.030029], [260.507334, 1024.908203], [260.757311, 1040.422485], [261.006944, 1052.170166], [261.257494, 1067.752808], [261.507318, 1079.557983], [261.757295, 1095.120728], [262.007463, 1106.912476], [262.256906, 1122.577515], [262.507379, 1134.186646], [262.757433, 1149.883179], [263.006761, 1161.492554], [263.257387, 1177.129028], [263.50725, 1188.759888], [263.75715, 1204.522339], [264.007623, 1216.029175], [264.257028, 1231.698608], [264.507349, 1243.386841], [264.757631, 1259.071655], [265.006845, 1270.544312], [265.257471, 1286.292358], [265.507105, 1297.889771], [265.757387, 1313.465942], [266.007593, 1325.187134], [266.257189, 1340.756226], [266.507509, 1352.456421], [266.757601, 1367.988892], [267.006815, 1379.701294], [267.25725, 1395.331909], [267.507227, 1406.932007], [267.757356, 1422.572388], [268.007372, 1434.136108], [268.2567, 1449.746704], [268.50744, 1461.275757], [268.757684, 1477.038696], [269.006861, 1488.459351], [269.257334, 1504.045532], [269.507273, 1515.690552], [269.757364, 1531.254272], [270.007456, 1542.91394], [270.256861, 1558.431519], [270.507486, 1570.077026], [270.75773, 1585.602173], [271.006983, 1597.332397], [271.257227, 1612.8302], [271.507166, 1624.602661], [271.757219, 1640.258667], [272.007616, 1651.894409], [272.256792, 1667.616577], [272.507494, 1679.2677], [272.757662, 1694.911499], [273.006799, 1706.729858], [273.257387, 1722.459351], [273.507173, 1734.20813], [273.757303, 1749.980347], [274.007623, 1761.80896], [274.256799, 1777.632202], [274.507501, 1789.421021], [274.75744, 1805.461548], [275.006769, 1817.116089], [275.257509, 1833.098511], [275.507067, 1844.87146], [275.757349, 1860.798218], [276.007631, 1872.818726], [276.256922, 1888.619263], [276.507738, 1900.654175], [276.757372, 1916.541382], [277.006967, 1928.619751], [277.257479, 1944.485962], [277.507074, 1956.638306], [277.757547, 1972.643677], [278.007524, 1984.637085], [278.256777, 2000.696655], [278.507555, 2012.713501], [278.757532, 2028.859741], [279.006899, 2040.898804], [279.257486, 2056.988281], [279.507082, 2069.102539], [279.757517, 2085.29248], [280.007646, 2097.562988], [280.256593, 2113.664062], [280.507639, 2125.980957], [280.757616, 2142.192383], [281.006868, 2154.535156], [281.257608, 2170.884277], [281.506861, 2183.211426], [281.757143, 2199.629883], [282.007425, 2212.152344], [282.256639, 2228.393555], [282.507265, 2241.056641], [282.757509, 2257.61377], [283.006571, 2270.249023], [283.257616, 2286.622559], [283.507059, 2299.391113], [283.757379, 2316.081543], [284.007814, 2328.799805], [284.256571, 2345.611816], [284.50754, 2358.452637], [284.757364, 2375.133789], [285.006426, 2388.111328], [285.257547, 2405.050293], [285.506914, 2418.149414], [285.757463, 2435.056641], [286.007707, 2448.061035], [286.256769, 2465.207031], [286.507662, 2478.276367], [286.757562, 2495.660156], [287.006624, 2508.848633], [287.257479, 2525.993652], [287.506883, 2539.394531], [287.757395, 2556.601562], [288.007601, 2570.078613], [288.256319, 2587.509277], [288.507593, 2600.885254], [288.757417, 2618.457031], [289.006746, 2632.058105], [289.257448, 2649.54541], [289.506967, 2663.168457], [289.757479, 2681.018555], [290.006998, 2694.625977], [290.256441, 2712.594238], [290.507791, 2726.294434], [290.757044, 2744.27002], [291.007059, 2758.307129], [291.257227, 2776.423828], [291.506822, 2790.497559], [291.757715, 2808.54834], [292.007158, 2822.947754], [292.25641, 2841.117187], [292.507646, 2855.615723], [292.757204, 2874.175293], [293.00699, 2888.668457], [293.257234, 2907.394043], [293.506983, 2921.967285], [293.757684, 2940.764648], [294.007547, 2955.61084], [294.256609, 2974.557129], [294.507578, 2989.666504], [294.757402, 3008.851074], [295.006883, 3023.855957], [295.257242, 3043.122559], [295.506952, 3058.595703], [295.757654, 3077.949707], [296.007631, 3093.593262], [296.256655, 3113.106934], [296.507547, 3128.864258], [296.757181, 3148.724121], [297.006777, 3164.496094], [297.257364, 3184.333496], [297.506578, 3200.461914], [297.757662, 3220.428223], [298.007334, 3236.770508], [298.256624, 3257.060059], [298.50744, 3273.340332], [298.756845, 3293.84082], [299.006822, 3310.248535], [299.25699, 3330.954102], [299.506586, 3347.804199], [299.757555, 3368.688965], [300.007036, 3385.443848], [300.256441, 3406.710449], [300.507639, 3423.666016], [300.757044, 3445.233398], [301.006906, 3462.583984], [301.257265, 3484.055176], [301.506708, 3501.868652], [301.75741, 3523.556641], [302.007273, 3541.65918], [302.256334, 3563.640625], [302.507456, 3581.986816], [302.757242, 3604.291992], [303.00699, 3622.917969], [303.25712, 3645.620605], [303.506563, 3664.383301], [303.757608, 3687.41748], [304.00728, 3706.543457], [304.25638, 3729.861328], [304.507616, 3749.258789], [304.757173, 3772.975586], [305.006769, 3792.70459], [305.256975, 3816.87793], [305.506761, 3836.771484], [305.757501, 3861.098633], [306.007135, 3881.727051], [306.256006, 3906.224609], [306.507242, 3927.152832], [306.756876, 3952.310059], [307.006624, 3973.406738], [307.256906, 3998.673828], [307.506235, 4020.36084], [307.757128, 4046.003418], [308.007143, 4068.144531], [308.256052, 4094.183594], [308.507326, 4116.676758], [308.756998, 4143.375], [309.006555, 4166.085937], [309.256723, 4193.455078], [309.506586, 4216.638184], [309.757364, 4244.004395], [310.006807, 4267.944824], [310.255983, 4295.854004], [310.507486, 4320.07666], [310.75712, 4348.86084], [311.006487, 4373.915039], [311.256883, 4402.96582], [311.506555, 4428.655273], [311.757067, 4458.27002], [312.007082, 4484.854004], [312.255686, 4515.246094], [312.50715, 4541.936035], [312.756937, 4573.075684], [313.006113, 4600.719727], [313.256586, 4632.455566], [313.506296, 4660.935547], [313.757189, 4693.465332], [314.007051, 4722.841309], [314.255579, 4756.562012], [314.507158, 4786.59375], [314.756868, 4820.96582], [315.005968, 4851.761719], [315.256403, 4887.206055], [315.506075, 4919.02832], [315.756967, 4955.479492], [316.006639, 4988.321289], [316.255167, 5025.898926], [316.506937, 5059.946289], [316.756647, 5098.475098], [317.005861, 5133.760742], [317.255876, 5173.31543], [317.505625, 5209.92041], [317.757128, 5250.793945], [318.006876, 5288.943848], [318.254907, 5331.289062], [318.506754, 5370.644531], [318.75696, 5414.602051], [319.005564, 5455.94043], [319.25577, 5501.380859], [319.505823, 5544.212891], [319.757059, 5591.436523], [320.006006, 5635.819824], [320.25419, 5685.346191], [320.506151, 5731.505859], [320.756433, 5783.373535], [321.005266, 5831.832031], [321.252802, 5885.831055], [321.476457, 5936.397949], [321.677454, 5987.70752], [321.85705, 6031.210937], [322.021311, 6074.248535], [322.158907, 6109.776855], [322.286165, 6143.467285], [322.387979, 6169.817871], [322.465418, 6193.82666], [322.533205, 6208.231934], [322.576807, 6222.145996], [322.597711, 6225.980957], [322.60763, 6227.273437], [322.668283, 6221.355469], [322.794931, 6228.822754], [322.90922, 6248.952148], [322.929094, 6273.858398], [322.950342, 6280.922852], [322.967623, 6285.711914], [322.979868, 6282.900391], [322.987383, 6281.447266], [322.992342, 6274.234863], [322.995241, 6269.831055], [322.99711, 6260.794434], [322.998064, 6255.466797], [322.99875, 6246.227539], [322.999056, 6240.991211], [322.999361, 6231.996094], [322.999666, 6227.307129], [322.999742, 6219.010742], [322.999819, 6214.929687], [322.999895, 6207.204102], [322.999895, 6203.682129], [322.999895, 6196.551758], [322.999895, 6193.493652], [322.999895, 6186.795898], [322.999971, 6184.177246], [323.000009, 6177.749512], [322.999895, 6175.503418], [322.999857, 6169.564453], [322.999971, 6167.640137], [322.999819, 6161.943848], [322.999933, 6160.241211], [322.999933, 6154.727539], [323.000009, 6153.291992], [322.999819, 6148.044922], [322.996958, 6146.787109], [322.980097, 6141.46582], [322.925737, 6137.133301], [322.841547, 6118.830078], [322.743433, 6093.608398], [322.63109, 6056.152344], [322.497385, 6016.044922], [322.343729, 5965.702637], [322.171686, 5913.027832], [321.977098, 5851.633301], [321.765764, 5788.497559], [321.532991, 5717.845703], [321.279733, 5646.79248], [321.006944, 5569.108398], [320.713785, 5491.931641], [320.401819, 5409.283203], [320.066507, 5327.785645], [319.714144, 5240.634766], [319.341677, 5156.92627], [318.948229, 5068.261719], [318.535364, 4983.019043], [318.102052, 4893.444824], [317.649477, 4806.966309], [317.194879, 4718.065918], [316.74711, 4634.690918], [316.297548, 4550.619141], [315.846575, 4472.839355], [315.396631, 4394.724609], [314.946726, 4323.611328], [314.496897, 4251.962891], [314.046457, 4185.705078], [313.596819, 4119.202637], [313.146646, 4057.828125], [312.696131, 3995.910645], [312.247103, 3938.742676], [311.796205, 3880.689453], [311.346109, 3827.213867], [310.8967, 3772.145508], [310.446413, 3722.348633], [309.99605, 3670.726562], [309.546678, 3623.290527], [309.095857, 3574.189941], [308.645914, 3529.155762], [308.196962, 3482.035156], [307.74576, 3439.652832], [307.296198, 3394.552246], [306.846216, 3353.680664], [306.396044, 3310.694336], [305.946138, 3271.54834], [305.4965, 3230.197754], [305.045488, 3192.563965], [304.596002, 3152.405762], [304.146173, 3116.560547], [303.695581, 3078.069824], [303.246439, 3043.272949], [302.795885, 3005.976562], [302.345865, 2972.086426], [301.896112, 2936.007812], [301.445711, 2903.761719], [300.995577, 2868.418945], [300.546167, 2837.181641], [300.095804, 2802.846191], [299.64567, 2772.55127], [299.196298, 2739.095215], [298.745363, 2709.616699], [298.295915, 2677.029297], [297.845896, 2648.013672], [297.395456, 2616.29248], [296.94578, 2588.043457], [296.496103, 2556.789551], [296.045511, 2529.42334], [295.595949, 2498.744629], [295.145929, 2471.938965], [294.695032, 2442.088867], [294.246156, 2415.577148], [293.795564, 2386.259277], [293.345468, 2360.266113], [292.896059, 2331.232422], [292.445772, 2306.028809], [291.995485, 2277.524414], [291.546076, 2252.766113], [291.095484, 2224.730957], [290.645464, 2200.403809], [290.196474, 2172.808594], [289.74531, 2148.904785], [289.295595, 2121.681641], [288.845804, 2098.166992], [288.395593, 2071.26416], [287.945612, 2047.892944], [287.495783, 2021.523315], [287.045267, 1998.410522], [286.595667, 1972.117065], [286.145876, 1949.474243], [285.695398, 1923.689087], [285.245836, 1901.114624], [284.795397, 1875.335327], [284.345491, 1853.004028], [283.895891, 1827.862183], [283.445566, 1805.745239], [282.995508, 1780.50769], [282.54587, 1758.910522], [282.095773, 1733.919312], [281.645448, 1712.529663], [281.195772, 1687.796265], [280.745485, 1666.649048], [280.295847, 1642.154663], [279.845674, 1621.070679], [279.395464, 1596.922729], [278.945368, 1576.036987], [278.495653, 1552.085083], [278.045328, 1531.36145], [277.595499, 1507.384644], [277.145822, 1486.997192], [276.695345, 1463.344116], [276.245783, 1442.876099], [275.795648, 1419.369507], [275.345667, 1399.03479], [274.895876, 1375.450073], [274.445398, 1355.450073], [273.99534, 1332.006958], [273.545702, 1312.121216], [273.095567, 1288.798218], [272.645395, 1268.889771], [272.195986, 1245.921997], [271.745355, 1226.314575], [271.295526, 1203.316772], [270.845506, 1183.796753], [270.395601, 1160.924683], [269.945581, 1141.40686], [269.495676, 1118.847534], [269.04558, 1099.410522], [268.59556, 1076.716187], [268.145998, 1057.630127], [267.695406, 1035.244873], [267.245577, 1015.988892], [266.795481, 993.445557], [266.345537, 974.306763], [265.895517, 952.012695], [265.44565, 932.952759], [264.995363, 910.733398], [264.545267, 891.869263], [264.095743, 869.778198], [263.645456, 850.796265], [263.195818, 828.61145], [262.745302, 809.807373], [262.29574, 787.86853], [261.845529, 769.286743], [261.395738, 747.292358], [260.945184, 728.612427], [260.495432, 706.957642], [260.045679, 688.392334], [259.595773, 666.562866], [259.145487, 648.181396], [258.695505, 626.456909], [258.245867, 607.959717], [257.795542, 586.426758], [257.34556, 568.021851], [0.0, 0.0], [0.0, 0.0], [0.0, 0.0], [0.0, 0.0], [0.0, 0.0], [0.0, 0.0], [0.0, 0.0], [0.0, 0.0], [0.0, 0.0], [0.0, 0.0], [0.0, 0.0], [0.0, 0.0], [0.0, 0.0], [0.0, 0.0], [0.0, 0.0], [0.0, 0.0], [0.0, 0.0], [0.0, 0.0], [0.0, 0.0], [0.0, 0.0], [0.0, 0.0], [0.0, 0.0]] ("all rows")
          }
          frame Enabled {
          }
        }
        n46 = Enqueue Element(queue=w214, element=w209, error in (no error)=w212) -> (error out=w213:errorcluster)  [unwired: 1 in, 2 out]
        n47 = call <vilib>:"Application Directory.vi"() -> ("Application Directory"=w171:path)
        n48 = Build Path(base path=w171, name or relative path=path "Data/Mini/Excel") -> (appended path=w174:path)
        n49 = Build Path(base path=w174, name or relative path=path "Tur Verileri") -> (appended path=w170:path)
        n50 = call <vilib>:"Check if File or Folder Exists.vi"("path"=w170) -> ("error out"=w202:errorcluster, "file or folder exists?"=w204:bool, "dup path"=w203:path)  [unwired: 8 in]
        n51 = for {
          N: 1 -> [_]
          shift-right: [w228] -> w187
          shift-left: string[] [] -> [w227]
          i -> [w223]
          w219 = "."
          n52 = Increment(x=w223) -> (x+1=w224:i32)
          n53 = Number To Decimal String(number=w224) -> (decimal integer string=w218:string)  [unwired: 1 in]
          n54 = call <vilib>:"Space Constant.vi"() -> ("String"=w221:string)
          n55 = Concatenate Strings(w218, w219, w221, "Kuvvet") -> (w225:string)
          n56 = Concatenate Strings(w218, w219, w221, "Pozisyon") -> (w226:string)
          n57 = Build Array (concatenate)(w227, w226, w225) -> (w228:string[])
        }
        n58 = case shown="False" w204 {
          tunnel: w203 -> [w238 w240]
          tunnel: [w237 w240] -> w183
          tunnel: w202 -> [w236 w239]
          tunnel: [w235 w239] -> w198
          frame False {
            n59 = Create Folder(path (use dialog)=w238, error in=w236) -> (created path=w237:path, error out=w235:errorcluster)  [unwired: 1 in, 1 out]
          }
          frame True {
          }
        }
        n60 = Get Date/Time In Seconds() -> (seconds since 1Jan1904=w206:timestamp)
        n61 = call <vilib>:"Check if File or Folder Exists.vi"("error in (no error)"=w198, "path"=w183) -> ("error out"=w199:errorcluster, "file or folder exists?"=w201:bool, "dup path"=w200:path)  [unwired: 7 in]
        n62 = Format Date/Time String(time format string (%c)="%y-%m-%d", seconds (now)=w206) -> (date/time string=w181:string)  [unwired: 1 in]
        n63 = call <vilib>:"Space Constant.vi"() -> ("String"=w182:string)
        n64 = case shown="False" w201 {
          tunnel: w200 -> [w232 w234]
          tunnel: [w231 w234] -> w197
          tunnel: w199 -> [w230 w233]
          tunnel: [w229 w233] -> w195
          frame False {
            n65 = Create Folder(path (use dialog)=w232, error in=w230) -> (created path=w231:path, error out=w229:errorcluster)  [unwired: 1 in, 1 out]
          }
          frame True {
          }
        }
        n66 = call <vilib>:"Space Constant.vi"() -> ("String"=w180:string)
        n67 = Concatenate Strings("Tarih" ("string"), w180, w181, w182, "Adet" ("string"), "_" ("string"), w167, ".csv" ("string")) -> (w177:string)
        n68 = Build Path(base path=w197, name or relative path=w177) -> (appended path=w192:path)
        n69 = Number To Fractional String(number=dbl[][] [[1.0, 1.0], [244.257944, 45.058472], [244.507425, 58.662598], [244.757021, 77.658325], [245.006311, 94.001465], [245.25667, 114.316162], [245.507105, 131.029785], [245.757044, 151.04895], [246.006906, 167.49231], [246.256769, 187.022217], [246.507318, 202.838623], [246.757372, 221.95752], [247.006471, 237.069092], [247.257021, 255.672485], [247.507189, 270.313477], [247.757128, 288.54126], [248.007219, 302.773437], [248.2567, 320.695068], [248.507364, 334.658569], [248.757532, 352.358887], [249.00667, 366.036377], [249.257448, 383.486328], [249.507044, 397.035278], [249.757326, 414.338745], [250.007417, 427.50415], [250.256822, 444.507324], [250.507562, 457.680054], [250.757463, 474.576172], [251.00683, 487.561768], [251.257379, 504.411011], [251.507013, 517.157349], [251.757181, 533.88916], [252.007463, 546.530029], [252.256868, 563.121338], [252.507532, 575.629883], [252.757318, 592.188599], [253.006723, 604.656616], [253.257387, 621.057129], [253.507326, 633.444458], [253.757112, 649.878906], [254.007547, 662.192505], [254.25699, 678.359985], [254.507463, 690.679443], [254.757402, 706.931396], [255.006807, 719.049927], [255.257395, 735.057617], [255.507257, 747.286377], [255.757273, 763.268311], [256.007631, 775.393555], [256.256883, 791.341064], [256.507433, 803.436523], [256.757486, 819.349731], [257.006853, 831.404297], [257.257326, 847.233398], [257.507189, 859.23291], [257.75728, 875.164185], [258.007601, 887.022461], [258.256853, 902.898071], [258.507364, 914.703979], [258.757532, 930.603638], [259.006784, 942.289917], [259.257372, 958.166626], [259.507234, 969.790161], [259.757402, 985.563843], [260.007379, 997.39856], [260.256746, 1013.030029], [260.507334, 1024.908203], [260.757311, 1040.422485], [261.006944, 1052.170166], [261.257494, 1067.752808], [261.507318, 1079.557983], [261.757295, 1095.120728], [262.007463, 1106.912476], [262.256906, 1122.577515], [262.507379, 1134.186646], [262.757433, 1149.883179], [263.006761, 1161.492554], [263.257387, 1177.129028], [263.50725, 1188.759888], [263.75715, 1204.522339], [264.007623, 1216.029175], [264.257028, 1231.698608], [264.507349, 1243.386841], [264.757631, 1259.071655], [265.006845, 1270.544312], [265.257471, 1286.292358], [265.507105, 1297.889771], [265.757387, 1313.465942], [266.007593, 1325.187134], [266.257189, 1340.756226], [266.507509, 1352.456421], [266.757601, 1367.988892], [267.006815, 1379.701294], [267.25725, 1395.331909], [267.507227, 1406.932007], [267.757356, 1422.572388], [268.007372, 1434.136108], [268.2567, 1449.746704], [268.50744, 1461.275757], [268.757684, 1477.038696], [269.006861, 1488.459351], [269.257334, 1504.045532], [269.507273, 1515.690552], [269.757364, 1531.254272], [270.007456, 1542.91394], [270.256861, 1558.431519], [270.507486, 1570.077026], [270.75773, 1585.602173], [271.006983, 1597.332397], [271.257227, 1612.8302], [271.507166, 1624.602661], [271.757219, 1640.258667], [272.007616, 1651.894409], [272.256792, 1667.616577], [272.507494, 1679.2677], [272.757662, 1694.911499], [273.006799, 1706.729858], [273.257387, 1722.459351], [273.507173, 1734.20813], [273.757303, 1749.980347], [274.007623, 1761.80896], [274.256799, 1777.632202], [274.507501, 1789.421021], [274.75744, 1805.461548], [275.006769, 1817.116089], [275.257509, 1833.098511], [275.507067, 1844.87146], [275.757349, 1860.798218], [276.007631, 1872.818726], [276.256922, 1888.619263], [276.507738, 1900.654175], [276.757372, 1916.541382], [277.006967, 1928.619751], [277.257479, 1944.485962], [277.507074, 1956.638306], [277.757547, 1972.643677], [278.007524, 1984.637085], [278.256777, 2000.696655], [278.507555, 2012.713501], [278.757532, 2028.859741], [279.006899, 2040.898804], [279.257486, 2056.988281], [279.507082, 2069.102539], [279.757517, 2085.29248], [280.007646, 2097.562988], [280.256593, 2113.664062], [280.507639, 2125.980957], [280.757616, 2142.192383], [281.006868, 2154.535156], [281.257608, 2170.884277], [281.506861, 2183.211426], [281.757143, 2199.629883], [282.007425, 2212.152344], [282.256639, 2228.393555], [282.507265, 2241.056641], [282.757509, 2257.61377], [283.006571, 2270.249023], [283.257616, 2286.622559], [283.507059, 2299.391113], [283.757379, 2316.081543], [284.007814, 2328.799805], [284.256571, 2345.611816], [284.50754, 2358.452637], [284.757364, 2375.133789], [285.006426, 2388.111328], [285.257547, 2405.050293], [285.506914, 2418.149414], [285.757463, 2435.056641], [286.007707, 2448.061035], [286.256769, 2465.207031], [286.507662, 2478.276367], [286.757562, 2495.660156], [287.006624, 2508.848633], [287.257479, 2525.993652], [287.506883, 2539.394531], [287.757395, 2556.601562], [288.007601, 2570.078613], [288.256319, 2587.509277], [288.507593, 2600.885254], [288.757417, 2618.457031], [289.006746, 2632.058105], [289.257448, 2649.54541], [289.506967, 2663.168457], [289.757479, 2681.018555], [290.006998, 2694.625977], [290.256441, 2712.594238], [290.507791, 2726.294434], [290.757044, 2744.27002], [291.007059, 2758.307129], [291.257227, 2776.423828], [291.506822, 2790.497559], [291.757715, 2808.54834], [292.007158, 2822.947754], [292.25641, 2841.117187], [292.507646, 2855.615723], [292.757204, 2874.175293], [293.00699, 2888.668457], [293.257234, 2907.394043], [293.506983, 2921.967285], [293.757684, 2940.764648], [294.007547, 2955.61084], [294.256609, 2974.557129], [294.507578, 2989.666504], [294.757402, 3008.851074], [295.006883, 3023.855957], [295.257242, 3043.122559], [295.506952, 3058.595703], [295.757654, 3077.949707], [296.007631, 3093.593262], [296.256655, 3113.106934], [296.507547, 3128.864258], [296.757181, 3148.724121], [297.006777, 3164.496094], [297.257364, 3184.333496], [297.506578, 3200.461914], [297.757662, 3220.428223], [298.007334, 3236.770508], [298.256624, 3257.060059], [298.50744, 3273.340332], [298.756845, 3293.84082], [299.006822, 3310.248535], [299.25699, 3330.954102], [299.506586, 3347.804199], [299.757555, 3368.688965], [300.007036, 3385.443848], [300.256441, 3406.710449], [300.507639, 3423.666016], [300.757044, 3445.233398], [301.006906, 3462.583984], [301.257265, 3484.055176], [301.506708, 3501.868652], [301.75741, 3523.556641], [302.007273, 3541.65918], [302.256334, 3563.640625], [302.507456, 3581.986816], [302.757242, 3604.291992], [303.00699, 3622.917969], [303.25712, 3645.620605], [303.506563, 3664.383301], [303.757608, 3687.41748], [304.00728, 3706.543457], [304.25638, 3729.861328], [304.507616, 3749.258789], [304.757173, 3772.975586], [305.006769, 3792.70459], [305.256975, 3816.87793], [305.506761, 3836.771484], [305.757501, 3861.098633], [306.007135, 3881.727051], [306.256006, 3906.224609], [306.507242, 3927.152832], [306.756876, 3952.310059], [307.006624, 3973.406738], [307.256906, 3998.673828], [307.506235, 4020.36084], [307.757128, 4046.003418], [308.007143, 4068.144531], [308.256052, 4094.183594], [308.507326, 4116.676758], [308.756998, 4143.375], [309.006555, 4166.085937], [309.256723, 4193.455078], [309.506586, 4216.638184], [309.757364, 4244.004395], [310.006807, 4267.944824], [310.255983, 4295.854004], [310.507486, 4320.07666], [310.75712, 4348.86084], [311.006487, 4373.915039], [311.256883, 4402.96582], [311.506555, 4428.655273], [311.757067, 4458.27002], [312.007082, 4484.854004], [312.255686, 4515.246094], [312.50715, 4541.936035], [312.756937, 4573.075684], [313.006113, 4600.719727], [313.256586, 4632.455566], [313.506296, 4660.935547], [313.757189, 4693.465332], [314.007051, 4722.841309], [314.255579, 4756.562012], [314.507158, 4786.59375], [314.756868, 4820.96582], [315.005968, 4851.761719], [315.256403, 4887.206055], [315.506075, 4919.02832], [315.756967, 4955.479492], [316.006639, 4988.321289], [316.255167, 5025.898926], [316.506937, 5059.946289], [316.756647, 5098.475098], [317.005861, 5133.760742], [317.255876, 5173.31543], [317.505625, 5209.92041], [317.757128, 5250.793945], [318.006876, 5288.943848], [318.254907, 5331.289062], [318.506754, 5370.644531], [318.75696, 5414.602051], [319.005564, 5455.94043], [319.25577, 5501.380859], [319.505823, 5544.212891], [319.757059, 5591.436523], [320.006006, 5635.819824], [320.25419, 5685.346191], [320.506151, 5731.505859], [320.756433, 5783.373535], [321.005266, 5831.832031], [321.252802, 5885.831055], [321.476457, 5936.397949], [321.677454, 5987.70752], [321.85705, 6031.210937], [322.021311, 6074.248535], [322.158907, 6109.776855], [322.286165, 6143.467285], [322.387979, 6169.817871], [322.465418, 6193.82666], [322.533205, 6208.231934], [322.576807, 6222.145996], [322.597711, 6225.980957], [322.60763, 6227.273437], [322.668283, 6221.355469], [322.794931, 6228.822754], [322.90922, 6248.952148], [322.929094, 6273.858398], [322.950342, 6280.922852], [322.967623, 6285.711914], [322.979868, 6282.900391], [322.987383, 6281.447266], [322.992342, 6274.234863], [322.995241, 6269.831055], [322.99711, 6260.794434], [322.998064, 6255.466797], [322.99875, 6246.227539], [322.999056, 6240.991211], [322.999361, 6231.996094], [322.999666, 6227.307129], [322.999742, 6219.010742], [322.999819, 6214.929687], [322.999895, 6207.204102], [322.999895, 6203.682129], [322.999895, 6196.551758], [322.999895, 6193.493652], [322.999895, 6186.795898], [322.999971, 6184.177246], [323.000009, 6177.749512], [322.999895, 6175.503418], [322.999857, 6169.564453], [322.999971, 6167.640137], [322.999819, 6161.943848], [322.999933, 6160.241211], [322.999933, 6154.727539], [323.000009, 6153.291992], [322.999819, 6148.044922], [322.996958, 6146.787109], [322.980097, 6141.46582], [322.925737, 6137.133301], [322.841547, 6118.830078], [322.743433, 6093.608398], [322.63109, 6056.152344], [322.497385, 6016.044922], [322.343729, 5965.702637], [322.171686, 5913.027832], [321.977098, 5851.633301], [321.765764, 5788.497559], [321.532991, 5717.845703], [321.279733, 5646.79248], [321.006944, 5569.108398], [320.713785, 5491.931641], [320.401819, 5409.283203], [320.066507, 5327.785645], [319.714144, 5240.634766], [319.341677, 5156.92627], [318.948229, 5068.261719], [318.535364, 4983.019043], [318.102052, 4893.444824], [317.649477, 4806.966309], [317.194879, 4718.065918], [316.74711, 4634.690918], [316.297548, 4550.619141], [315.846575, 4472.839355], [315.396631, 4394.724609], [314.946726, 4323.611328], [314.496897, 4251.962891], [314.046457, 4185.705078], [313.596819, 4119.202637], [313.146646, 4057.828125], [312.696131, 3995.910645], [312.247103, 3938.742676], [311.796205, 3880.689453], [311.346109, 3827.213867], [310.8967, 3772.145508], [310.446413, 3722.348633], [309.99605, 3670.726562], [309.546678, 3623.290527], [309.095857, 3574.189941], [308.645914, 3529.155762], [308.196962, 3482.035156], [307.74576, 3439.652832], [307.296198, 3394.552246], [306.846216, 3353.680664], [306.396044, 3310.694336], [305.946138, 3271.54834], [305.4965, 3230.197754], [305.045488, 3192.563965], [304.596002, 3152.405762], [304.146173, 3116.560547], [303.695581, 3078.069824], [303.246439, 3043.272949], [302.795885, 3005.976562], [302.345865, 2972.086426], [301.896112, 2936.007812], [301.445711, 2903.761719], [300.995577, 2868.418945], [300.546167, 2837.181641], [300.095804, 2802.846191], [299.64567, 2772.55127], [299.196298, 2739.095215], [298.745363, 2709.616699], [298.295915, 2677.029297], [297.845896, 2648.013672], [297.395456, 2616.29248], [296.94578, 2588.043457], [296.496103, 2556.789551], [296.045511, 2529.42334], [295.595949, 2498.744629], [295.145929, 2471.938965], [294.695032, 2442.088867], [294.246156, 2415.577148], [293.795564, 2386.259277], [293.345468, 2360.266113], [292.896059, 2331.232422], [292.445772, 2306.028809], [291.995485, 2277.524414], [291.546076, 2252.766113], [291.095484, 2224.730957], [290.645464, 2200.403809], [290.196474, 2172.808594], [289.74531, 2148.904785], [289.295595, 2121.681641], [288.845804, 2098.166992], [288.395593, 2071.26416], [287.945612, 2047.892944], [287.495783, 2021.523315], [287.045267, 1998.410522], [286.595667, 1972.117065], [286.145876, 1949.474243], [285.695398, 1923.689087], [285.245836, 1901.114624], [284.795397, 1875.335327], [284.345491, 1853.004028], [283.895891, 1827.862183], [283.445566, 1805.745239], [282.995508, 1780.50769], [282.54587, 1758.910522], [282.095773, 1733.919312], [281.645448, 1712.529663], [281.195772, 1687.796265], [280.745485, 1666.649048], [280.295847, 1642.154663], [279.845674, 1621.070679], [279.395464, 1596.922729], [278.945368, 1576.036987], [278.495653, 1552.085083], [278.045328, 1531.36145], [277.595499, 1507.384644], [277.145822, 1486.997192], [276.695345, 1463.344116], [276.245783, 1442.876099], [275.795648, 1419.369507], [275.345667, 1399.03479], [274.895876, 1375.450073], [274.445398, 1355.450073], [273.99534, 1332.006958], [273.545702, 1312.121216], [273.095567, 1288.798218], [272.645395, 1268.889771], [272.195986, 1245.921997], [271.745355, 1226.314575], [271.295526, 1203.316772], [270.845506, 1183.796753], [270.395601, 1160.924683], [269.945581, 1141.40686], [269.495676, 1118.847534], [269.04558, 1099.410522], [268.59556, 1076.716187], [268.145998, 1057.630127], [267.695406, 1035.244873], [267.245577, 1015.988892], [266.795481, 993.445557], [266.345537, 974.306763], [265.895517, 952.012695], [265.44565, 932.952759], [264.995363, 910.733398], [264.545267, 891.869263], [264.095743, 869.778198], [263.645456, 850.796265], [263.195818, 828.61145], [262.745302, 809.807373], [262.29574, 787.86853], [261.845529, 769.286743], [261.395738, 747.292358], [260.945184, 728.612427], [260.495432, 706.957642], [260.045679, 688.392334], [259.595773, 666.562866], [259.145487, 648.181396], [258.695505, 626.456909], [258.245867, 607.959717], [257.795542, 586.426758], [257.34556, 568.021851], [0.0, 0.0], [0.0, 0.0], [0.0, 0.0], [0.0, 0.0], [0.0, 0.0], [0.0, 0.0], [0.0, 0.0], [0.0, 0.0], [0.0, 0.0], [0.0, 0.0], [0.0, 0.0], [0.0, 0.0], [0.0, 0.0], [0.0, 0.0], [0.0, 0.0], [0.0, 0.0], [0.0, 0.0], [0.0, 0.0], [0.0, 0.0], [0.0, 0.0], [0.0, 0.0], [0.0, 0.0]] ("all rows"), precision (6)=i16 6) -> (F-format string=w185:string[][])  [unwired: 2 in]
        n70 = Open/Create/Replace File(file path (use dialog)=w192, error in=w195, operation (0:open)=T11."open or create") -> (refnum out=w194:refnum<file>, error out=w193:errorcluster)  [unwired: 3 in, 1 out]
        n71 = Build Array (concatenate)(w187, w185) -> (w186:string[][])
        n72 = Close File(refnum=w194, error in=w193) -> (error out=w191:errorcluster)  [unwired: 1 out]
        n73 = call-poly <vilib>:"Write Delimited Spreadsheet.vi"("file path (dialog if empty)"=w192, "2D data"=w186, "error in (no error)"=w191, "delimiter (\\t)"=";" ("delimiter (\\t)")) -> ()  [unwired: 10 in, 2 out]
      }
      frame "Compare" {
        # "Action 2 - Send an \"Update Display\" message indicating which button was pressed. Note that a string is sent as the Message Data along with the \"Update Display\" message."
        n74 = property on="Languages" class="Ring (strict)"() -> ("Value"=w241:u16)  [unwired: 2 in, 2 out]
        n75 = case shown="2" w241 {
          tunnel: ["Karşılaştır" ("L10n_Action 2 Pressed") "Compare" ("L10n_Action 2 Pressed") "Vergleichen" ("L10n_Action 2 Pressed")] -> w242
          frame 0, Default {
          }
          frame 1 {
          }
          frame 2 {
          }
        }
        n76 = Bundle By Name(cluster=T10 {"Message"="", "Message Data"=variant} ("Message Cluster"), "Message"="Update Display", "Message Data"=w242) -> (w247:T10)
        n77 = flat-sequence {
          frame #0 {
            n78 = call <vilib>:"Application Directory.vi"() -> ("Application Directory"=w258:path)
            n79 = Build Path(base path=w258, name or relative path=path "Data/Mini/Referans") -> (appended path=w256:path)
            n80 = List Folder(path=w256) -> (filenames=w261:string[])  [unwired: 3 in, 3 out]
            n81 = for {
              tunnel: w261 -> [w262] mode=indexing
              shift-right: [w266] -> w260
              shift-left: string[] [] -> [w267]
              n82 = String Length(string=w262) -> (length=w264:i32)
              n83 = Subtract(x=w264, y=4) -> (x-y=w263:i32)
              n84 = Match Pattern(string=w262, regular expression="", offset (0)=w263) -> (before substring=w268:string, after substring=w269:string)  [unwired: 2 out]
              n85 = case shown="\".csv\"" w269 {
                tunnel: w268 -> [_ w272]
                tunnel: w267 -> [w271 w274]
                tunnel: [w271 w273] -> w266
                frame "False", Default {
                }
                frame ".csv" {
                  n86 = Build Array (concatenate)(w274, w272) -> (w273:string[])
                }
              }
            }
            n87 = property on="Referans Veriler" class="LstBox (strict)"("Item Names"=w260) -> ()  [unwired: 2 in, 2 out]
          }
          frame #1 {
            n88 = property on="Display Message" class="Str"("Blinking"=FALSE, "Text.BGColor"=u32 5140359 ("Text.Text Colors:BG Color"), "Text.TextColor"=u32 16777225 ("Text.Text Colors:Text Color")) -> ()  [unwired: 2 in, 2 out]
          }
        }
        n89 = Enqueue Element(queue=w252, element=w247, error in (no error)=w250) -> (error out=w251:errorcluster)  [unwired: 1 in, 2 out]
      }
      frame "Alarms" {
        # "Action 2 - Send an \"Update Display\" message indicating which button was pressed. Note that a string is sent as the Message Data along with the \"Update Display\" message."
        n90 = property on="Languages" class="Ring (strict)"(error in=w279) -> ("Value"=w280:u16)  [unwired: 1 in, 2 out]
        n91 = case shown="2" w280 {
          tunnel: ["Alarmlar" ("L10n_Action 2 Pressed") "Alarms" ("L10n_Action 2 Pressed") "Alarm" ("L10n_Action 2 Pressed")] -> w278
          frame 0, Default {
          }
          frame 1 {
          }
          frame 2 {
          }
        }
        n92 = Bundle By Name(cluster=T10 {"Message"="", "Message Data"=variant} ("Message Cluster"), "Message"="Update Display", "Message Data"=w278) -> (w285:T10)
        n93 = Enqueue Element(queue=w290, element=w285, error in (no error)=w288) -> (error out=w289:errorcluster)  [unwired: 1 in, 2 out]
      }
      frame "Manuel" {
        # "Action 2 - Send an \"Update Display\" message indicating which button was pressed. Note that a string is sent as the Message Data along with the \"Update Display\" message."
        n94 = property on="Languages" class="Ring (strict)"(error in=w295) -> ("Value"=w296:u16)  [unwired: 1 in, 2 out]
        n95 = case shown="2" w296 {
          tunnel: ["Manuel" ("L10n_Action 2 Pressed") "Manual" ("L10n_Action 2 Pressed") "Manual" ("L10n_Action 2 Pressed")] -> w294
          frame 0, Default {
          }
          frame 1 {
          }
          frame 2 {
          }
        }
        n96 = Bundle By Name(cluster=T10 {"Message"="", "Message Data"=variant} ("Message Cluster"), "Message"="Update Display", "Message Data"=w294) -> (w301:T10)
        n97 = Enqueue Element(queue=w306, element=w301, error in (no error)=w304) -> (error out=w305:errorcluster)  [unwired: 1 in, 2 out]
      }
      frame "Calibration" {
        # "Action 2 - Send an \"Update Display\" message indicating which button was pressed. Note that a string is sent as the Message Data along with the \"Update Display\" message."
        n98 = property on="Languages" class="Ring (strict)"() -> ("Value"=w311:u16)  [unwired: 2 in, 2 out]
        n99 = case shown="0, Default" w311 {
          tunnel: ["Kalibrasyon" ("L10n_Action 2 Pressed") "Calibration" ("L10n_Action 2 Pressed") "Kalibrierung" ("L10n_Action 2 Pressed")] -> w310
          frame 0, Default {
          }
          frame 1 {
          }
          frame 2 {
          }
        }
        n100 = Bundle By Name(cluster=T10 {"Message"="", "Message Data"=variant} ("Message Cluster"), "Message"="Update Display", "Message Data"=w310) -> (w316:T10)
        n101 = Enqueue Element(queue=w321, element=w316, error in (no error)=w319) -> (error out=w320:errorcluster)  [unwired: 1 in, 2 out]
      }
      frame "Exit" {
        # "Exit - Exit the application. Since this message was sent as a priority message (i.e., it was placed at the front of the queue), any cleanup code should run here, since the loop is about to stop. Any other messages in the queue will not be handled."
        n102 = property on="Languages" class="Ring (strict)"() -> ("Value"=w326:u16)  [unwired: 2 in, 2 out]
        n103 = case shown="0, Default" w326 {
          tunnel: ["ÇIKIŞ" ("L10n_Action 2 Pressed") "EXIT" ("L10n_Action 2 Pressed") "AUSGANG" ("L10n_Action 2 Pressed")] -> w325
          frame 0, Default {
          }
          frame 1 {
          }
          frame 2 {
          }
        }
        n104 = Release Queue(queue=w334, error in (no error)=w331) -> (error out=w332:errorcluster)  [unwired: 1 in, 2 out]
        n105 = local write "Display Message"(w325) -> ()
      }
      frame "Continue" {
        # "Action 2 - Send an \"Update Display\" message indicating which button was pressed. Note that a string is sent as the Message Data along with the \"Update Display\" message."
        n106 = property on="Languages" class="Ring (strict)"() -> ("Value"=w339:u16)  [unwired: 2 in, 2 out]
        n107 = case shown="2" w339 {
          tunnel: ["Devam Et" ("L10n_Action 2 Pressed") "Continue" ("L10n_Action 2 Pressed") "Fortsetzen" ("L10n_Action 2 Pressed")] -> w338
          frame 0, Default {
          }
          frame 1 {
          }
          frame 2 {
          }
        }
        n108 = Bundle By Name(cluster=T10 {"Message"="", "Message Data"=variant} ("Message Cluster"), "Message"="Update Display", "Message Data"=w338) -> (w344:T10)
        n109 = Enqueue Element(queue=w349, element=w344, error in (no error)=w347) -> (error out=w348:errorcluster)  [unwired: 1 in, 2 out]
      }
      frame "Mold Recipe Search" {
        # "Action 2 - Send an \"Update Display\" message indicating which button was pressed. Note that a string is sent as the Message Data along with the \"Update Display\" message."
        n110 = flat-sequence {
          tunnel: [w372] -> w360
          tunnel: w360 -> [w378]
          tunnel: w358 -> [w377]
          tunnel: [w376] -> w357
          frame #0 {
            n111 = property on="moldSelection" class="LstBox (strict)"() -> ("Item Names"=w375:string[])  [unwired: 2 in, 2 out]
            n112 = property on="searchRecipe" class="Str"() -> ("Value"=w373:string)  [unwired: 2 in, 2 out]
            n113 = Search 1D Array(1D array=w375, element=w373) -> (index of element=w374:i32)  [unwired: 1 in]
            n114 = Greater Or Equal To 0?(x=w374) -> (x >= 0?=w372:bool)
            n115 = Select(t=w374, s=w372, f=nan) -> (s? t:f=w370:dbl)
            n116 = property on="moldSelection" class="LstBox (strict)"("Value"=w370) -> ()  [unwired: 2 in, 2 out]
          }
          frame #1 {
            n117 = case shown="True" w378 {
              tunnel: w377 -> [w381 w401]
              tunnel: [w379 w398] -> w376
              frame False {
                n118 = Replace Array Subset(array=w381, new element=0 ("new element/subarray"), index=2) -> (w379:i32[])
                n119 = property on="pieceNo" class="Str"("Value"="" ("pieceNo")) -> ()  [unwired: 2 in, 2 out]
                n120 = property on="serialNo" class="Str"("Value"="" ("serialNo")) -> ()  [unwired: 2 in, 2 out]
                n121 = property on="KALIP BİLGİLERİ" class="Clust (strict)"("Value"=T12 {"Parça No"="", "Seri No"="", "Müşteri"="", "Kalıp No"="", "Kuvvet Limiti [kN]"="", "Kuvvet Limiti [kN] 2"=""} ("KALIP BİLGİLERİ")) -> ()  [unwired: 2 in, 2 out]
                n122 = property on="KONTROL PARAM" class="Clust (strict)"("Value"=T3 {"Kuvvet Limit"="", "Grafik Limit"=""} ("KONTROL PARAM")) -> ()  [unwired: 2 in, 2 out]
                n123 = property on="HAREKET PROFİLİ" class="Clust (strict)"("Value"=T4 {"TDC"=0.0, "S1"=0.0, "P1"=0.0, "S2"=0.0, "BDC"=0.0, "S3"=0.0, "Bekleme Süresi"=0.0} ("HAREKET PROFİLİ")) -> ()  [unwired: 2 in, 2 out]
              }
              frame True {
                n124 = Replace Array Subset(array=w401, new element=1 ("new element/subarray"), index=2) -> (w398:i32[])
                n125 = property on="moldSelection" class="LstBox (strict)"() -> ("Item Names"=w397:string[], "Value"=w396:i32)  [unwired: 2 in, 2 out]
                n126 = call "recipeWriteToIndicator.vi"("Value"=w396, "Item Names"=w397) -> ("Cluster"=w395:T13)  [unwired: 9 in]
                n127 = Unbundle(w395) -> ("KALIP BİLGİLERİ 2"=w394:T12, "Parça No"=w393:string, "Seri No"=w392:string, "KALIP BİLGİLERİ"=w391:T14, "HAREKET PROFİLİ"=w390:T4, "new picture"=w389:picture, "picture index"=w388:dbl)
                n128 = property on="KALIP BİLGİLERİ" class="Clust (strict)"("Value"=w394) -> ()  [unwired: 2 in, 2 out]
                n129 = local write "pieceNo"(w393) -> ()
                n130 = local write "serialNo"(w392) -> ()
                n131 = property on="KONTROL PARAM" class="Clust (strict)"("Value"=w391) -> ()  [unwired: 2 in, 2 out]
                n132 = property on="HAREKET PROFİLİ" class="Clust (strict)"("Value"=w390) -> ()  [unwired: 2 in, 2 out]
                n133 = property on="2D Picture" class="Pict"("Value"=w389) -> ()  [unwired: 2 in, 2 out]
                n134 = property on="Image" class="LstBox (strict)"("Value"=w388) -> ()  [unwired: 2 in, 2 out]
              }
            }
          }
        }
        n135 = property on="Languages" class="Ring (strict)"() -> ("Value"=w354:u16)  [unwired: 2 in, 2 out]
        n136 = case shown="0, Default" w354 {
          tunnel: ["Reçete Ara" ("L10n_Action 2 Pressed") "Recipe Search" ("L10n_Action 2 Pressed") "Rezeptsuche" ("L10n_Action 2 Pressed")] -> w353
          frame 0, Default {
          }
          frame 1 {
          }
          frame 2 {
          }
        }
        n137 = Bundle By Name(cluster=T10 {"Message"="", "Message Data"=variant} ("Message Cluster"), "Message"="Update Display", "Message Data"=w353) -> (w361:T10)
        n138 = Enqueue Element(queue=w366, element=w361, error in (no error)=w364) -> (error out=w365:errorcluster)  [unwired: 1 in, 2 out]
      }
      frame "Registration Page" {
        # "Action 2 - Send an \"Update Display\" message indicating which button was pressed. Note that a string is sent as the Message Data along with the \"Update Display\" message."
        n139 = property on="Languages" class="Ring (strict)"() -> ("Value"=w403:u16)  [unwired: 2 in, 2 out]
        n140 = case shown="2" w403 {
          tunnel: ["Kayıt Sayfası" ("L10n_Action 2 Pressed") "Registration Page" ("L10n_Action 2 Pressed") "Registrierungsseite" ("L10n_Action 2 Pressed")] -> w402
          frame 0, Default {
          }
          frame 1 {
          }
          frame 2 {
          }
        }
        n141 = Replace Array Subset(array=w412, new element #1=1 ("new element/subarray"), index #1=3 ("index"), new element #2=0 ("new element/subarray"), index #2=4 ("index")) -> (w407:i32[])
        n142 = Bundle By Name(cluster=T10 {"Message"="", "Message Data"=variant} ("Message Cluster"), "Message"="Update Display", "Message Data"=w402) -> (w413:T10)
        n143 = Enqueue Element(queue=w418, element=w413, error in (no error)=w416) -> (error out=w417:errorcluster)  [unwired: 1 in, 2 out]
      }
      frame "Test Edit" {
        # "Action 2 - Send an \"Update Display\" message indicating which button was pressed. Note that a string is sent as the Message Data along with the \"Update Display\" message."
        n144 = property on="Languages" class="Ring (strict)"() -> ("Value"=w423:u16)  [unwired: 2 in, 2 out]
        n145 = case shown="0, Default" w423 {
          tunnel: ["Testi Düzenle" ("L10n_Action 2 Pressed") "Test Edit" ("L10n_Action 2 Pressed") "Testbearbeitung" ("L10n_Action 2 Pressed")] -> w422
          frame 0, Default {
          }
          frame 1 {
          }
          frame 2 {
          }
        }
        n146 = Bundle By Name(cluster=T10 {"Message"="", "Message Data"=variant} ("Message Cluster"), "Message"="Update Display", "Message Data"=w422) -> (w428:T10)
        n147 = Enqueue Element(queue=w433, element=w428, error in (no error)=w431) -> (error out=w432:errorcluster)  [unwired: 1 in, 2 out]
      }
      frame "New Recipe" {
        # "Action 2 - Send an \"Update Display\" message indicating which button was pressed. Note that a string is sent as the Message Data along with the \"Update Display\" message."
        n148 = property on="Languages" class="Ring (strict)"() -> ("Value"=w438:u16)  [unwired: 2 in, 2 out]
        n149 = case shown="0, Default" w438 {
          tunnel: ["Yeni Reçete" ("L10n_Action 2 Pressed") "New Recipe" ("L10n_Action 2 Pressed") "Neues Rezept" ("L10n_Action 2 Pressed")] -> w437
          frame 0, Default {
          }
          frame 1 {
          }
          frame 2 {
          }
        }
        n150 = flat-sequence {
          tunnel: w451 -> [w471]
          tunnel: [w477] -> w444
          frame #0 {
            n151 = property on="Image" class="LstBox (strict)"() -> ("Item Names"=w463:string[], "Value"=w462:i32)  [unwired: 2 in, 2 out]
            n152 = property on="KALIP BİLGİLERİ" class="Clust (strict)"() -> ("Value"=w468:T2)  [unwired: 2 in, 2 out]
            n153 = property on="KONTROL PARAM" class="Clust (strict)"() -> ("Value"=w466:T3)  [unwired: 2 in, 2 out]
            n154 = property on="HAREKET PROFİLİ" class="Clust (strict)"() -> ("Value"=w469:T4)  [unwired: 2 in, 2 out]
            n155 = Index Array(array=w463, index=w462) -> (element=w461:string)
            n156 = Unbundle By Name(w468) -> ("Parça No"=w470:string)
            n157 = Flatten To XML(6:w468) -> (2:w465:string)
            n158 = Flatten To XML(6:w466) -> (2:w464:string)
            n159 = Flatten To XML(6:w469) -> (2:w476:string)
            n160 = Flatten To XML(6:w461) -> (2:w460:string)
            n161 = call <vilib>:"Application Directory.vi"() -> ("Application Directory"=w473:path)
            n162 = Build Path(base path=w473, name or relative path=path "Data/Receipt") -> (appended path=w472:path)
            n163 = Concatenate Strings(w465, w464, w476, w460) -> (w475:string)
            n164 = call "MiniPNewXmlBuild.vi"("error in"=w471, "XMLinput"=w475, "Ürün İsmi"=w470, "Path"=w472) -> ("error out"=w477:errorcluster, "Kalıparr"=w467:string[])  [unwired: 6 in]
            n165 = property on="moldSelection" class="LstBox (strict)"("Item Names"=w467) -> ()  [unwired: 2 in, 2 out]
          }
        }
        n166 = Bundle By Name(cluster=T10 {"Message"="", "Message Data"=variant} ("Message Cluster"), "Message"="Update Display", "Message Data"=w437) -> (w452:T10)
        n167 = Enqueue Element(queue=w456, element=w452, error in (no error)=w455) -> (error out=w443:errorcluster)  [unwired: 1 in, 2 out]
        n168 = Merge Errors(w444, w443) -> (w442:errorcluster)
        n169 = property on="Test Pages Tab" class="TabCtl (strict)"() -> ("Value"=w448:enum32{"0", "1", "2", "3", "4", "5"})  [unwired: 2 in, 2 out]
        n170 = property on="Test Button Tab" class="TabCtl (strict)"() -> ("Value"=w447:enum32{"0", "1", "2", "3", "4", "5"})  [unwired: 2 in, 2 out]
        n171 = Replace Array Subset(array=w445, new element #1=w448, index #1=4 ("index"), new element #2=w447, index #2=5 ("index")) -> (w446:i32[])
      }
      frame "Recipe Save" {
        # "Action 2 - Send an \"Update Display\" message indicating which button was pressed. Note that a string is sent as the Message Data along with the \"Update Display\" message."
        n172 = call <vilib>:"Application Directory.vi"() -> ("Application Directory"=w499:path)
        n173 = property on="KALIP BİLGİLERİ" class="Clust (strict)"() -> ("Value"=w491:T2)  [unwired: 2 in, 2 out]
        n174 = Unbundle By Name(w491) -> ("Parça No"=w490:string)
        n175 = Build Path(base path=w499, name or relative path=path "Data/Receipt") -> (appended path=w495:path)
        n176 = List Folder(path=w495) -> (filenames=w494:string[])  [unwired: 3 in, 3 out]
        n177 = Concatenate Strings(w490, "", ".xml") -> (w489:string)
        n178 = property on="Languages" class="Ring (strict)"() -> ("Value"=w479:u16)  [unwired: 2 in, 2 out]
        n179 = case shown="1" w479 {
          tunnel: ["Reçete Kaydet" ("L10n_Action 2 Pressed") "Save Recipe" ("L10n_Action 2 Pressed") "Rezept Speichern" ("L10n_Action 2 Pressed")] -> w478
          frame 0, Default {
          }
          frame 1 {
          }
          frame 2 {
          }
        }
        n180 = Search 1D Array(1D array=w494, element=w489) -> (index of element=w496:i32)  [unwired: 1 in]
        n181 = Greater Or Equal To 0?(x=w496) -> (x >= 0?=w493:bool)
        n182 = case shown="True" w493 {
          tunnel: w495 -> [_ w510]
          tunnel: w494 -> [_ w509]
          frame False {
          }
          frame True {
            n183 = flat-sequence {
              tunnel: w510 -> [w519]
              tunnel: w509 -> [w532]
              frame #0 {
                n184 = property on="KALIP BİLGİLERİ" class="Clust (strict)"() -> ("Value"=w521:T2)  [unwired: 2 in, 2 out]
                n185 = property on="KONTROL PARAM" class="Clust (strict)"() -> ("Value"=w517:T3)  [unwired: 2 in, 2 out]
                n186 = property on="HAREKET PROFİLİ" class="Clust (strict)"() -> ("Value"=w522:T4)  [unwired: 2 in, 2 out]
                n187 = property on="Image" class="LstBox (strict)"() -> ("Item Names"=w514:string[], "Value"=w513:i32)  [unwired: 2 in, 2 out]
                n188 = Index Array(array=w514, index=w513) -> (element=w512:string)
                n189 = Unbundle By Name(w521) -> ("Parça No"=w520:string)
                n190 = Concatenate Strings(w520, "" ("string"), ".xml" ("string")) -> (w528:string)
                n191 = call <vilib>:"Trim Whitespace.vi"("string"=w528) -> ("trimmed string"=w529:string)  [unwired: 1 in]
                n192 = Flatten To XML(6:w521) -> (2:w523:string)
                n193 = Flatten To XML(6:w517) -> (2:w515:string)
                n194 = Flatten To XML(6:w522) -> (2:w516:string)
                n195 = Flatten To XML(6:w512) -> (2:w511:string)
                n196 = Build Path(base path=w519, name or relative path=w529) -> (appended path=w530:path)
                n197 = call <vilib>:"Check if File or Folder Exists.vi"("path"=w530) -> ("error out"=w526:errorcluster, "dup path"=w527:path)  [unwired: 8 in, 1 out]
                n198 = Concatenate Strings(w523, w515, w516, w511) -> (w518:string)
                n199 = call-poly <vilib>:"Write to XML File.vi"("error in (no error)"=w526, "XML Input"=w518, "XML File Path"=w527) -> ()  [unwired: 6 in, 3 out]
              }
              frame #1 {
                n200 = for {
                  tunnel: w532 -> [w534] mode=indexing
                  shift-right: [w538] -> w533
                  shift-left: string[] [] -> [w539]
                  n201 = String Length(string=w534) -> (length=w537:i32)
                  n202 = Subtract(x=w537, y=4) -> (x-y=w535:i32)
                  n203 = Match Pattern(string=w534, regular expression="", offset (0)=w535) -> (before substring=w540:string, after substring=w541:string)  [unwired: 2 out]
                  n204 = case shown="\".xml\"" w541 {
                    tunnel: w540 -> [_ w544]
                    tunnel: w539 -> [w543 w546]
                    tunnel: [w543 w545] -> w538
                    frame "False", Default {
                    }
                    frame ".xml" {
                      n205 = Build Array (concatenate)(w546, w544) -> (w545:string[])
                    }
                  }
                }
                n206 = property on="moldSelection" class="LstBox (strict)"("Item Names"=w533) -> ()  [unwired: 2 in, 2 out]
              }
            }
          }
        }
        n207 = property on="Test Pages Tab" class="TabCtl (strict)"() -> ("Value"=w485:enum32{"0", "1", "2", "3", "4", "5"})  [unwired: 2 in, 2 out]
        n208 = property on="Test Button Tab" class="TabCtl (strict)"() -> ("Value"=w484:enum32{"0", "1", "2", "3", "4", "5"})  [unwired: 2 in, 2 out]
        n209 = Replace Array Subset(array=w488, new element #1=w485, index #1=4 ("index"), new element #2=w484, index #2=5 ("index")) -> (w483:i32[])
        n210 = Bundle By Name(cluster=T10 {"Message"="", "Message Data"=variant} ("Message Cluster"), "Message"="Update Display", "Message Data"=w478) -> (w501:T10)
        n211 = Enqueue Element(queue=w505, element=w501, error in (no error)=w504) -> (error out=w492:errorcluster)  [unwired: 1 in, 2 out]
      }
      frame "Recipe Delete" {
        # "Action 2 - Send an \"Update Display\" message indicating which button was pressed. Note that a string is sent as the Message Data along with the \"Update Display\" message."
        n212 = flat-sequence {
          frame #0 {
            n213 = property on="moldSelection" class="LstBox (strict)"() -> ("Item Names"=w563:string[], "Value"=w562:i32)  [unwired: 2 in, 2 out]
            n214 = Index Array(array=w563, index=w562) -> (element=w569:string)
            n215 = Concatenate Strings(w569, ".xml" ("string")) -> (w567:string)
            n216 = call <vilib>:"Application Directory.vi"() -> ("Application Directory"=w565:path)
            n217 = Build Path(base path=w565, name or relative path=path "Data/Receipt") -> (appended path=w564:path)
            n218 = Build Path(base path=w564, name or relative path=w567) -> (appended path=w570:path)
            n219 = Delete(path (use dialog)=w570) -> ()  [unwired: 4 in, 3 out]
          }
          frame #1 {
            n220 = call <vilib>:"Application Directory.vi"() -> ("Application Directory"=w573:path)
            n221 = Build Path(base path=w573, name or relative path=path "Data/Receipt") -> (appended path=w572:path)
            n222 = List Folder(path=w572) -> (filenames=w576:string[])  [unwired: 3 in, 3 out]
            n223 = for {
              tunnel: w576 -> [w577] mode=indexing
              shift-right: [w581] -> w571
              shift-left: string[] [] -> [w582]
              n224 = String Length(string=w577) -> (length=w579:i32)
              n225 = Subtract(x=w579, y=4) -> (x-y=w578:i32)
              n226 = Match Pattern(string=w577, regular expression="", offset (0)=w578) -> (before substring=w583:string, after substring=w584:string)  [unwired: 2 out]
              n227 = case shown="\".xml\"" w584 {
                tunnel: w583 -> [_ w587]
                tunnel: w582 -> [w586 w589]
                tunnel: [w586 w588] -> w581
                frame "False", Default {
                }
                frame ".xml" {
                  n228 = Build Array (concatenate)(w589, w587) -> (w588:string[])
                }
              }
            }
            n229 = property on="moldSelection" class="LstBox (strict)"("Item Names"=w571) -> ()  [unwired: 2 in, 2 out]
          }
        }
        n230 = property on="Languages" class="Ring (strict)"() -> ("Value"=w548:u16)  [unwired: 2 in, 2 out]
        n231 = case shown="0, Default" w548 {
          tunnel: ["Reçete Sil" ("L10n_Action 2 Pressed") "Delete Recipe" ("L10n_Action 2 Pressed") "Rezept Löschen" ("L10n_Action 2 Pressed")] -> w547
          frame 0, Default {
          }
          frame 1 {
          }
          frame 2 {
          }
        }
        n232 = Bundle By Name(cluster=T10 {"Message"="", "Message Data"=variant} ("Message Cluster"), "Message"="Update Display", "Message Data"=w547) -> (w553:T10)
        n233 = Enqueue Element(queue=w558, element=w553, error in (no error)=w556) -> (error out=w557:errorcluster)  [unwired: 1 in, 2 out]
      }
      frame "Recipe Send" {
        # "Action 2 - Send an \"Update Display\" message indicating which button was pressed. Note that a string is sent as the Message Data along with the \"Update Display\" message."
        n234 = property on="Languages" class="Ring (strict)"() -> ("Value"=w591:u16)  [unwired: 2 in, 2 out]
        n235 = case shown="0, Default" w591 {
          tunnel: ["Reçete Gönder" ("L10n_Action 2 Pressed") "Send Recipe" ("L10n_Action 2 Pressed") "Rezept Senden" ("L10n_Action 2 Pressed")] -> w590
          frame 0, Default {
          }
          frame 1 {
          }
          frame 2 {
          }
        }
        n236 = Bundle By Name(cluster=T10 {"Message"="", "Message Data"=variant} ("Message Cluster"), "Message"="Update Display", "Message Data"=w590) -> (w596:T10)
        n237 = Enqueue Element(queue=w601, element=w596, error in (no error)=w599) -> (error out=w600:errorcluster)  [unwired: 1 in, 2 out]
      }
      frame "Add Referance" {
        # "Action 2 - Send an \"Update Display\" message indicating which button was pressed. Note that a string is sent as the Message Data along with the \"Update Display\" message."
        n238 = flat-sequence {
          tunnel: w611 -> [w630]
          tunnel: [w624] -> w610
          tunnel: [w623] -> w606
          tunnel: w605 -> [w622]
          frame #0 {
            n239 = property on="Referans Veriler" class="LstBox (strict)"() -> ("Item Names"=w627:string[], "Value"=w626:i32)  [unwired: 2 in, 2 out]
            n240 = Build Array (concatenate)(w630, w626) -> (w624:i32[])
            n241 = call "MiniPCompareData.vi"("all rows 3"=w622, "Alt Limit"="Alt Limit", "Referans Veriler"=w627, "Veri Aralığı"=w624) -> ("all rows"=w623:dbl[][], "CompareXY"=→"Comparexy":T6)  [unwired: 6 in]
            n242 = Array Size(array=w624) -> (size(s)=w631:i32)
            n243 = Number To Decimal String(number=w631) -> (decimal integer string=→"Grafik Sayısı":string)  [unwired: 1 in]
          }
        }
        n244 = property on="Languages" class="Ring (strict)"() -> ("Value"=w608:u16)  [unwired: 2 in, 2 out]
        n245 = case shown="0, Default" w608 {
          tunnel: ["Referans Ekle" ("L10n_Action 2 Pressed") "Add Referance" ("L10n_Action 2 Pressed") "Füge Referenz Hinzu" ("L10n_Action 2 Pressed")] -> w607
          frame 0, Default {
          }
          frame 1 {
          }
          frame 2 {
          }
        }
        n246 = Bundle By Name(cluster=T10 {"Message"="", "Message Data"=variant} ("Message Cluster"), "Message"="Update Display", "Message Data"=w607) -> (w613:T10)
        n247 = Enqueue Element(queue=w618, element=w613, error in (no error)=w616) -> (error out=w617:errorcluster)  [unwired: 1 in, 2 out]
      }
      frame "Delete Reference" {
        # "Action 2 - Send an \"Update Display\" message indicating which button was pressed. Note that a string is sent as the Message Data along with the \"Update Display\" message."
        n248 = flat-sequence {
          tunnel: w638 -> [w651]
          tunnel: [w651] -> w636
          tunnel: w635 -> [w649]
          tunnel: [w652] -> w634
          frame #0 {
            n249 = property on="Referans Veriler" class="LstBox (strict)"() -> ("Value"=w654:i32)  [unwired: 2 in, 2 out]
            n250 = call "MiniCompareDelete.vi"("Value"=w654, "output array 2"=w649, "Veri Aralığı"=w651) -> ("output array 3"=w652:dbl[][], "CompareXY 2"=w653:T6)  [unwired: 7 in]
            n251 = property on="Comparexy" class="XYGraph (strict)"("Value"=w653) -> ()  [unwired: 2 in, 2 out]
            n252 = Array Size(array=w651) -> (size(s)=w655:i32)
            n253 = Number To Decimal String(number=w655) -> (decimal integer string=w650:string)  [unwired: 1 in]
            n254 = property on="Grafik Sayısı" class="Str"("Value"=w650) -> ()  [unwired: 2 in, 2 out]
          }
        }
        n255 = property on="Languages" class="Ring (strict)"() -> ("Value"=w633:u16)  [unwired: 2 in, 2 out]
        n256 = case shown="0, Default" w633 {
          tunnel: ["Referans Sil" ("L10n_Action 2 Pressed") "Delete Referance" ("L10n_Action 2 Pressed") "Referenz Löschen" ("L10n_Action 2 Pressed")] -> w632
          frame 0, Default {
          }
          frame 1 {
          }
          frame 2 {
          }
        }
        n257 = Bundle By Name(cluster=T10 {"Message"="", "Message Data"=variant} ("Message Cluster"), "Message"="Update Display", "Message Data"=w632) -> (w640:T10)
        n258 = Enqueue Element(queue=w645, element=w640, error in (no error)=w643) -> (error out=w644:errorcluster)  [unwired: 1 in, 2 out]
      }
      frame "Update Display" {
        n259 = Variant To Data(error in=w664, type="", Variant=w663) -> (data=→"Display Message":string, error out=w662:errorcluster)
      }
      frame Default {
        # "The Default case only runs if there is a message that isn't defined in any of the other cases. Generate an error if this occurs."
        n260 = xnode "Error Ring"("parameter 0"=w671) -> ("error out"=w669:errorcluster)
        n261 = call <vilib>:"Simple Error Handler.vi"("error in (no error)"=w669) -> ()  [unwired: 4 in, 5 out]
      }
    }
    n262 = Index Array(array=w31, index #1=0 ("index")) -> (element #1=w32:i32, element #2=w29:i32, element #3=w28:i32, element #4=w27:i32, element #5=w26:i32, element #6=w25:i32)  [unwired: 5 in]
    n263 = property on="General Tab" class="TabCtl (strict)"("Val(Sgnl)"=w32) -> ()  [unwired: 2 in, 2 out]
    n264 = property on="General Pages Tab" class="TabCtl (strict)"("Val(Sgnl)"=w29) -> ()  [unwired: 2 in, 2 out]
    n265 = property on="Mold Choice Tab" class="TabCtl (strict)"("Val(Sgnl)"=w28) -> ()  [unwired: 2 in, 2 out]
    n266 = property on="Test Button General" class="TabCtl (strict)"("Val(Sgnl)"=w27) -> ()  [unwired: 2 in, 2 out]
    n267 = property on="Test Pages Tab" class="TabCtl (strict)"("Val(Sgnl)"=w26) -> ()  [unwired: 2 in, 2 out]
    n268 = property on="Test Button Tab" class="TabCtl (strict)"("Val(Sgnl)"=w25) -> ()  [unwired: 2 in, 2 out]
  }
  n269 = while {
    stop <- w748 stop-if-true
    n270 = control-ref of="bt_startHydraulicSystem"() -> (w713:refnum<vi>)
    n271 = control-ref of="bt_stopHydraulicSystem"() -> (w714:refnum<vi>)
    n272 = control-ref of="bt_testCall"() -> (w715:refnum<vi>)
    n273 = control-ref of="Display Message"() -> (w716:refnum<vi>)
    n274 = control-ref of="Pozisyon (Position)"() -> (w717:refnum<vi>)
    n275 = control-ref of="Kuvvet (Force)"() -> (w718:refnum<vi>)
    n276 = control-ref of="bt_testStart"() -> (w721:refnum<vi>)
    n277 = control-ref of="bt_testPause"() -> (w719:refnum<vi>)
    n278 = control-ref of="bt_testStop"() -> (w720:refnum<vi>)
    n279 = control-ref of="pieceNo"() -> (w727:refnum<vi>)
    n280 = control-ref of="bt_graphLimited"() -> (w722:refnum<vi>)
    n281 = control-ref of="bt_newRecipe"() -> (w723:refnum<vi>)
    n282 = control-ref of="bt_imageUpload"() -> (w724:refnum<vi>)
    n283 = control-ref of="bt_motionProfile"() -> (w725:refnum<vi>)
    n284 = control-ref of="bt_recipeSave"() -> (w728:refnum<vi>)
    n285 = control-ref of="bt_controlParameters"() -> (w729:refnum<vi>)
    n286 = control-ref of="bt_recipeSend"() -> (w730:refnum<vi>)
    n287 = control-ref of="bt_moldInformation"() -> (w745:refnum<vi>)
    n288 = control-ref of="bt_recipeDelete"() -> (w731:refnum<vi>)
    n289 = control-ref of="bt_registrationPage"() -> (w732:refnum<vi>)
    n290 = control-ref of="bt_alarms"() -> (w733:refnum<vi>)
    n291 = control-ref of="bt_reportExcel"() -> (w734:refnum<vi>)
    n292 = control-ref of="bt_compare"() -> (w735:refnum<vi>)
    n293 = control-ref of="bt_testEdit"() -> (w736:refnum<vi>)
    n294 = control-ref of="serialNo"() -> (w737:refnum<vi>)
    n295 = control-ref of="bt_exit"() -> (w744:refnum<vi>)
    n296 = control-ref of="bt_calibration"() -> (w746:refnum<vi>)
    n297 = control-ref of="Pres Tur"() -> (w738:refnum<vi>)
    n298 = control-ref of="Kuvvet Limiti [kN]"() -> (w739:refnum<vi>)
    n299 = control-ref of="Kalıp No"() -> (w740:refnum<vi>)
    n300 = control-ref of="Müşteri"() -> (w741:refnum<vi>)
    n301 = control-ref of="Seri No"() -> (w742:refnum<vi>)
    n302 = control-ref of="Parça No"() -> (w743:refnum<vi>)
    n303 = control-ref of="Kuvvet Limit"() -> (w712:refnum<vi>)
    n304 = control-ref of="Grafik Limit"() -> (w711:refnum<vi>)
    n305 = control-ref of="Pozisyon"() -> (w710:refnum<vi>)
    n306 = control-ref of="Hız"() -> (w709:refnum<vi>)
    n307 = control-ref of="Bekleme Süresi"() -> (w708:refnum<vi>)
    n308 = control-ref of="Image"() -> (w707:refnum<vi>)
    n309 = control-ref of="tur"() -> (w706:refnum<vi>)
    n310 = control-ref of="Hız"() -> (w705:refnum<vi>)
    n311 = control-ref of="anlıkKuvvet"() -> (w704:refnum<vi>)
    n312 = control-ref of="Kuvvet"() -> (w703:refnum<vi>)
    n313 = control-ref of="MaxPozisyon"() -> (w702:refnum<vi>)
    n314 = control-ref of="MinPozisyon"() -> (w701:refnum<vi>)
    n315 = control-ref of="MaxPozisyon"() -> (w700:refnum<vi>)
    n316 = control-ref of="MinPozisyon"() -> (w699:refnum<vi>)
    n317 = control-ref of="poliTestCheckbox"() -> (w698:refnum<vi>)
    n318 = control-ref of="Referans Veriler"() -> (w697:refnum<vi>)
    n319 = control-ref of="Grafik Sayısı"() -> (w696:refnum<vi>)
    n320 = control-ref of="Alt Limit"() -> (w695:refnum<vi>)
    n321 = control-ref of="addReferance"() -> (w694:refnum<vi>)
    n322 = control-ref of="graphicReset"() -> (w693:refnum<vi>)
    n323 = control-ref of="deleteReferance"() -> (w692:refnum<vi>)
    n324 = Build Array(w713, w714, w715, w716, w717, w718, w721, w719, w720, w727, w722, w723, w724, w725, w728, w729, w730, w745, w731, w732, w733, w734, w735, w736, w737, w744, w746, w738, w739, w740, w741, w742, w743, w712, w711, w710, w709, w708, w707, w706, w705, w704, w703, w702, w701, w700, w699, w698, w697, w696, w695, w694, w693, w692) -> (w691:refnum<vi>[])
    n325 = case shown="1" "Languages" {
      tunnel: [string[] ["Sistem Başlat", "Sistem Durdur", "Test Çağır", "DURUM BİLGİSİ", "Pozisyon", "Kuvvet", "Test Başlat", "Test Durdur", "Test Bitir", "Parça No", "Grafik Sınırlayıcı", "Yeni Kayıt", "Resim Yükle", "Hareket Profili", "Kaydet", "Kontrol Parametreleri", "Çalışmaya Gönder", "Kalıp Bilgileri", "Sil", "Kayıt Sayfası", "Alarmlar", "Rapor", "Karşılaştır", "Testi Düzenle", "Seri No", "ÇIKIŞ", "Kalibrasyon", "Pres Tur", "Kuvvet Limiti [kN]", "Kalıp No", "Müşteri", "Seri No", "Parça No", "Kuvvet Limit", "Grafik Limit", "Pozisyon", "Hız", "Bekleme Süresi", "Resim Seç", "Pozisyon", "Hız", "Bekleme", "Kuvvet", "Max Pozisyon", "Min Pozisyon", "Max Kuvvet", "Min Kuvvet", "Çoklu Test", "Referans Veriler", "Grafik Sayısı", "Alt Limit", "Grafik Ekle", "Grafik Reset", "Sil"] ("appended array") string[] ["Start System", "Stop System", "Call Test", "DISPLAY MESSAGE", "Position", "Force", "Start Test", "Stop Test", "Finish Test", "Part No", "Graph Delimiter", "New Registration", "Upload Picture", "Motion Profile", "Save", "Control Parameters", "Send to Run", "Mold Information", "Delete", "Registration Page", "Alarms", "Report", "Compare", "Edit Test", "Serial No", "EXIT", "Calibration", "Press Round", "Force Limit [kN]", "Mold No", "Customer", "Serial No", "Part No", "Force Limit", "Graphic Limit", "Position", "Velocity", "Standby Time", "Select Image", "Position", "Velocity", "Wait", "Force", "Max Position", "Min Position", "Max Force", "Min Force", "Multiple Testing", "Reference Data", "Charts' Number", "Lower Limit", "Add Graph", "Reset Graph", "Delete"] ("appended array") string[] ["System Starten", "System Stoppen", "Anruftest", "NACHRICHT ANZEIGEN", "Position", "Gewalt", "Test Starten", "Test Stoppen", "Test Beenden", "Teil Nr", "Diagrammbegrenzer", "Neue Registrierung", "Bild Hochladen", "Bewegungsprofil", "Speichern", "Regelparameter", "Zum Laufen Schicken", "Schimmel Informationen", "Löschen", "Registrierungsseite", "Alarm", "Prüfbericht", "Vergleichen", "Prüfung Bearbeiten", "Seriennummer", "AUSGANG", "Kalibrierung", "Runde Drücken", "Limit Erzwingen", "Muster", "Kunde", "Seriennummer", "Teil Nr", "Limit Erzwingen", "Grafiklimit", "Position", "Geschwindigkeit", "Standby-Zeit", "Bild Auswahlen", "Position", "Geschwindigkeit", "Warte ab", "Gewalt", "Maximale Position", "Mindestposition", "Maximalkraft", "Mindestkraft", "Mehrfaches Testen", "Vergleichsdaten", "Nummer der Charts", "Untere Grenze", "Grafik Hinzufügen", "Grafik Zurücksetzen", "Löschen"] ("appended array")] -> w726
      frame 0, Default {
        # "Turkish"
      }
      frame 1 {
        # "English"
      }
      frame 2 {
        # "German"
      }
    }
    n326 = for {
      tunnel: w726 -> [w757] mode=indexing
      tunnel: w691 -> [w756] mode=indexing
      n327 = property class="Ctl"(reference=w756, "Caption.Text"=w757) -> ()  [unwired: 1 in, 2 out]
    }
    n328 = Boolean To (0,1)(Boolean="Bits") -> (0, 1=w688:i16[])
    n329 = Number To Decimal String(number=w688) -> (decimal integer string=w687:string[])  [unwired: 1 in]
    n330 = disable-structure shown="Disabled" {
      frame Disabled {
        # "message data için dil\nseçeneği"
        n331 = property on="Languages" class="Ring (strict)"() -> ("Value"=w752:u16)  [unwired: 2 in, 2 out]
        n332 = case shown="1" w752 {
          tunnel: ["Karşılaştır" ("L10n_Action 2 Pressed") "Compare" ("L10n_Action 2 Pressed") "Vergleichen" ("L10n_Action 2 Pressed")] -> _
          frame 0, Default {
          }
          frame 1 {
          }
          frame 2 {
          }
        }
      }
      frame Enabled {
      }
    }
    n333 = Insert Into Array(array=string[] [], new element=w687) -> (w686:string[])  [unwired: 1 in]
    n334 = Build Array(string[] ["Table top switch", "Table reference switch", "Table bottom switch", "Pump is running", "Pump motor error", "Circulation motor error", "Fan motor error", "Up to the park", "Operating button is selected as an adjustment mode", "Operating button is selected as a manual mode", "Operating button is selected as an auto mode", "P filter is clogged", "R filter is clogged", "Suction valve  switch", "Oil-Level switch", "Phase OK switch", "Valve S1", "Valve S2", "Valve S3", "Valve S4", "Valve S5", "Valve S6", "Valve S7", "Valve S8", "Pump is started", "Circulation motor is started", "Fan motor is started", "Green Light", "Red Light", "Yellow Light", "Light Reset"] ("subarray"), w686) -> (w685:string[][])
    n335 = Transpose 2D Array(2D array=w685) -> (transposed array=w682:string[][])
    "Table Control 2" <- w682
    n336 = Index Array(array=w682, index (col)=0 ("index")) -> (element=w681:string[])  [unwired: 1 in]
    n337 = Array Size(array=w681) -> (size(s)=w679:i32)
    n338 = for {
      N: w679 -> [_]
      tunnel: [w749] -> w680 mode=indexing
      i -> [w751]
      n339 = Increment(x=w751) -> (x+1=w750:i32)
      n340 = Number To Decimal String(number=w750) -> (decimal integer string=w749:string)  [unwired: 1 in]
    }
    n341 = property on="Table Control 2" class="Tbl (strict)"("Row Headers[]"=w680) -> ()  [unwired: 2 in, 2 out]
    n342 = local read "bt_exit"() -> (w748:bool)
  }
  n343 = property on="KALIP BİLGİLERİ" class="Clust (strict)"() -> ("Value"=→"KALIP BİLGİLERİ-ÇALIŞMAs":T2)  [unwired: 2 in, 2 out]
  n344 = call <vilib>:"Application Directory.vi"() -> ("Application Directory"=w7:path)
  n345 = Build Path(base path=w7, name or relative path=path "Data/Image") -> (appended path=w5:path)
  n346 = disable-structure shown="Disabled" {
    frame Disabled {
      (unwired) i32[] [1, 1, 1, 0, 0]
      n347 = property on="General Tab" class="TabCtl (strict)" props=["Val(Sgnl)"]() -> ()  [unwired: 3 in, 2 out]
      n348 = property on="General Pages Tab" class="TabCtl (strict)" props=["Val(Sgnl)"]() -> ()  [unwired: 3 in, 2 out]
      n349 = property on="Mold Choice Tab" class="TabCtl (strict)" props=["Val(Sgnl)"]() -> ()  [unwired: 3 in, 2 out]
      n350 = property on="Test Button Tab" class="TabCtl (strict)" props=["Val(Sgnl)"]() -> ()  [unwired: 3 in, 2 out]
      n351 = property on="Test Pages Tab" class="TabCtl (strict)" props=["Val(Sgnl)"]() -> ()  [unwired: 3 in, 2 out]
      n352 = property on="Color Box" class="ColBox"("Visible"=TRUE) -> ()  [unwired: 2 in, 2 out]
    }
    frame Enabled {
    }
  }
  n353 = while {
    tunnel: w15 -> [w768]
    tunnel: [w765] -> w17
    shift-right: [w762] -> _
    shift-left: w5 -> [w763]
    stop <- w767 stop-if-true
    # "Event Handling Loop"
    n354 = event shown="[10] \"bt_Manuel\": Value Change" {
      selector: _ -> [_ _ _ _ _ _ _ _ _ _ _ _ _ _ _ _ _ _ _ _ _ _ _ _ _ _ _ _ _ _ _]
      dyn-events: _ -> [_ _ _ _ _ _ _ _ _ _ _ _ _ _ _ _ _ _ _ _ _ _ _ _ _ _ _ _ _ _ _]
      timeout: _ -> [_ _ _ _ _ _ _ _ _ _ _ _ _ _ _ _ _ _ _ _ _ _ _ _ _ _ _ _ _ _ _]
      tunnel: [_ _ _ _ _ _ _ _ _ _ _ _ TRUE _ _ _ _ _ _ _ _ _ _ _ _ _ _ _ _ _ _] -> w767
      tunnel: w768 -> [w771 w774 w777 w780 w783 w786 w789 w792 w795 w798 w801 w804 w808 w811 w822 w839 w842 w863 w865 w867 w873 w875 w893 w902 w906 w909 w911 w922 w935 w976 w979]
      tunnel: [w770 w773 w776 w779 w782 w785 w788 w791 w794 w797 w800 w803 w807 w810 w821 w838 w841 _ _ _ _ _ _ _ w905 w908 w910 w921 _ w975 w978] -> w764
      tunnel: [_ _ _ _ _ _ _ _ _ _ _ _ _ _ _ _ _ w863 w865 w867 w873 w875 w893 w902 _ _ _ _ w935 _ _] -> w766
      tunnel: w763 -> [_ _ _ _ _ _ _ _ _ _ _ _ _ _ _ _ _ _ _ _ _ w877 _ _ _ _ _ _ _ _ _]
      tunnel: [_ _ _ _ _ _ _ _ _ _ _ _ _ _ _ _ _ _ _ _ _ w876 _ _ _ _ _ _ _ _ _] -> w762
      event "bt_home": Value Change {
        # "Enqueue an \"Action 1\" message."
        n355 = event-data() -> ()  [unwired: 1 in, 1 out]
        n356 = Enqueue Element(queue=w771, element=T10 {"Message"="Home", "Message Data"=variant}) -> (error out=w770:errorcluster)  [unwired: 2 in, 2 out]
      }
      event "bt_startHydraulicSystem": Value Change {
        # "Enqueue an \"Action 1\" message."
        n357 = event-data() -> ()  [unwired: 1 in, 1 out]
        n358 = Enqueue Element(queue=w774, element=T10 {"Message"="Hydraulic Start", "Message Data"=variant}) -> (error out=w773:errorcluster)  [unwired: 2 in, 2 out]
      }
      event "bt_stopHydraulicSystem": Value Change {
        # "Enqueue an \"Action 2\" message."
        n359 = event-data() -> ()  [unwired: 1 in, 6 out]
        n360 = Enqueue Element(queue=w777, element=T10 {"Message"="Hydraulic Stop", "Message Data"=variant}) -> (error out=w776:errorcluster)  [unwired: 2 in, 2 out]
      }
      event "bt_testCall": Value Change {
        # "Enqueue an \"Action 2\" message."
        n361 = event-data() -> ()  [unwired: 1 in, 6 out]
        n362 = Enqueue Element(queue=w780, element=T10 {"Message"="Test Call", "Message Data"=variant}) -> (error out=w779:errorcluster)  [unwired: 2 in, 2 out]
      }
      event "bt_testStart": Value Change {
        # "Enqueue an \"Action 2\" message."
        n363 = event-data() -> ()  [unwired: 1 in, 6 out]
        n364 = Enqueue Element(queue=w783, element=T10 {"Message"="Test Start", "Message Data"=variant}) -> (error out=w782:errorcluster)  [unwired: 2 in, 2 out]
      }
      event "bt_testPause": Value Change {
        # "Enqueue an \"Action 2\" message."
        n365 = event-data() -> ()  [unwired: 1 in, 6 out]
        n366 = Enqueue Element(queue=w786, element=T10 {"Message"="Test Pause", "Message Data"=variant}) -> (error out=w785:errorcluster)  [unwired: 2 in, 2 out]
      }
      event "bt_testStop": Value Change {
        # "Enqueue an \"Action 2\" message."
        n367 = event-data() -> ()  [unwired: 1 in, 6 out]
        n368 = Enqueue Element(queue=w789, element=T10 {"Message"="Test Stop", "Message Data"=variant}) -> (error out=w788:errorcluster)  [unwired: 2 in, 2 out]
      }
      event "bt_reportExcel": Value Change {
        # "Enqueue an \"Action 2\" message."
        n369 = event-data() -> ()  [unwired: 1 in, 6 out]
        n370 = Enqueue Element(queue=w792, element=T10 {"Message"="Report Excel", "Message Data"=variant}) -> (error out=w791:errorcluster)  [unwired: 2 in, 2 out]
      }
      event "bt_compare": Value Change {
        # "Enqueue an \"Action 2\" message."
        n371 = event-data() -> ()  [unwired: 1 in, 6 out]
        n372 = Enqueue Element(queue=w795, element=T10 {"Message"="Compare", "Message Data"=variant}) -> (error out=w794:errorcluster)  [unwired: 2 in, 2 out]
      }
      event "bt_alarms": Value Change {
        # "Enqueue an \"Action 2\" message."
        n373 = event-data() -> ()  [unwired: 1 in, 6 out]
        n374 = Enqueue Element(queue=w798, element=T10 {"Message"="Alarms", "Message Data"=variant}) -> (error out=w797:errorcluster)  [unwired: 2 in, 2 out]
      }
      event "bt_Manuel": Value Change {
        # "Enqueue an \"Action 2\" message."
        n375 = event-data() -> ()  [unwired: 1 in, 6 out]
        n376 = Enqueue Element(queue=w801, element=T10 {"Message"="Manuel", "Message Data"=variant}) -> (error out=w800:errorcluster)  [unwired: 2 in, 2 out]
      }
      event "bt_calibration": Value Change {
        # "Enqueue an \"Action 2\" message."
        n377 = event-data() -> ()  [unwired: 1 in, 6 out]
        n378 = Enqueue Element(queue=w804, element=T10 {"Message"="Calibration", "Message Data"=variant}) -> (error out=w803:errorcluster)  [unwired: 2 in, 2 out]
      }
      event "bt_exit": Value Change {
        # "Enqueue an \"Exit\" message. Note that the Enqueue Element At Opposite End function is used to place this priority \"Exit\" message at the front of the queue ahead of all other messages."
        n379 = event-data() -> ()  [unwired: 1 in, 1 out]
        n380 = Enqueue Element At Opposite End(queue=w808, element=T10 {"Message"="Exit", "Message Data"=variant}) -> (error out=w807:errorcluster)  [unwired: 2 in, 2 out]
      }
      event "bt_continue": Value Change {
        # "Enqueue an \"Exit\" message. Note that the Enqueue Element At Opposite End function is used to place this priority \"Exit\" message at the front of the queue ahead of all other messages."
        n381 = event-data() -> ()  [unwired: 1 in, 1 out]
        n382 = Enqueue Element(queue=w811, element=T10 {"Message"="Continue", "Message Data"=variant}) -> (error out=w810:errorcluster)  [unwired: 2 in, 2 out]
      }
      event "bt_moldRecipeSearch": Value Change {
        # "recepeSend butonunu reçete seçili \ndeğil iken de aktif eder"
        # "Enqueue an \"Exit\" message. Note that the Enqueue Element At Opposite End function is used to place this priority \"Exit\" message at the front of the queue ahead of all other messages."
        n383 = event-data() -> ()  [unwired: 1 in, 1 out]
        n384 = Enqueue Element(queue=w822, element=T10 {"Message"="Mold Recipe Search", "Message Data"=variant}) -> (error out=w821:errorcluster)  [unwired: 2 in, 2 out]
        n385 = property on="moldSelection" class="LstBox (strict)"() -> ("Item Names"=w818:string[], "Value"=w819:i32)  [unwired: 2 in, 2 out]
        n386 = Index Array(array=w818, index=w819) -> (element=w817:string)
        n387 = Equal?(x=w817, y="") -> (x = y?=w816:bool)
        n388 = Select(t=T15."Disabled and Grayed Out" ("Disabled"), s=w816, f=T15."Enabled" ("Disabled")) -> (s? t:f=w815:T15)
        n389 = property on="bt_recipeSend" class="Bool"("DisabledEnum"=w815) -> ()  [unwired: 2 in, 2 out]
      }
      event "bt_registrationPage": Value Change {
        # "recepeSend butonunu reçete seçili \ndeğil iken de aktif eder"
        # "Enqueue an \"Exit\" message. Note that the Enqueue Element At Opposite End function is used to place this priority \"Exit\" message at the front of the queue ahead of all other messages."
        n390 = event-data() -> ()  [unwired: 1 in, 1 out]
        n391 = Enqueue Element(queue=w839, element=T10 {"Message"="Registration Page", "Message Data"=variant}) -> (error out=w838:errorcluster)  [unwired: 2 in, 2 out]
        n392 = property on="moldSelection" class="LstBox (strict)"() -> ("Item Names"=w829:string[], "Value"=w830:i32)  [unwired: 2 in, 2 out]
        n393 = Index Array(array=w829, index=w830) -> (element=w828:string)
        n394 = Equal?(x=w828, y="") -> (x = y?=w827:bool)
        n395 = Select(t=T15."Disabled and Grayed Out" ("Disabled"), s=w827, f=T15."Enabled" ("Disabled")) -> (s? t:f=w826:T15)
        n396 = property on="bt_recipeSend" class="Bool"("DisabledEnum"=w826) -> ()  [unwired: 2 in, 2 out]
        n397 = property on="pieceNo" class="Str"("Value"="" ("pieceNo")) -> ()  [unwired: 2 in, 2 out]
        n398 = property on="serialNo" class="Str"("Value"="" ("serialNo")) -> ()  [unwired: 2 in, 2 out]
        n399 = property on="KALIP BİLGİLERİ" class="Clust (strict)"("Value"=T12 {"Parça No"="", "Seri No"="", "Müşteri"="", "Kalıp No"="", "Kuvvet Limiti [kN]"="", "Kuvvet Limiti [kN] 2"=""} ("KALIP BİLGİLERİ")) -> ()  [unwired: 2 in, 2 out]
        n400 = property on="KONTROL PARAM" class="Clust (strict)"("Value"=T3 {"Kuvvet Limit"="", "Grafik Limit"=""} ("KONTROL PARAM")) -> ()  [unwired: 2 in, 2 out]
        n401 = property on="HAREKET PROFİLİ" class="Clust (strict)"("Value"=T4 {"TDC"=0.0, "S1"=0.0, "P1"=0.0, "S2"=0.0, "BDC"=0.0, "S3"=0.0, "Bekleme Süresi"=0.0} ("HAREKET PROFİLİ")) -> ()  [unwired: 2 in, 2 out]
        n402 = property on="moldSelection" class="LstBox (strict)"("Value"=nan) -> ()  [unwired: 2 in, 2 out]
      }
      event "bt_testEdit": Value Change {
        # "Enqueue an \"Action 2\" message."
        n403 = event-data() -> ()  [unwired: 1 in, 1 out]
        n404 = disable-structure shown="Disabled" {
          frame Disabled {
            n405 = call <vilib>:"Application Directory.vi"() -> ("Application Directory"=w847:path)
            n406 = Build Path(base path=w847, name or relative path=path "Data/Receipt") -> (appended path=w848:path)
            n407 = call "searchRecipe.vi"("search string"="searchRecipe", "XML File Path"=w848) -> ("outFileNames"=w849:string[])  [unwired: 9 in]
            n408 = for {
              tunnel: w849 -> [w850] mode=indexing
              shift-right: [w854] -> w843
              shift-left: string[] [] -> [w855]
              n409 = String Length(string=w850) -> (length=w852:i32)
              n410 = Subtract(x=w852, y=4) -> (x-y=w851:i32)
              n411 = Match Pattern(string=w850, regular expression="", offset (0)=w851) -> (before substring=w856:string, after substring=w857:string)  [unwired: 2 out]
              n412 = case shown="\".xml\"" w857 {
                tunnel: w856 -> [_ w860]
                tunnel: w855 -> [w859 w862]
                tunnel: [w859 w861] -> w854
                frame "False", Default {
                }
                frame ".xml" {
                  n413 = Build Array (concatenate)(w862, w860) -> (w861:string[])
                }
              }
            }
            n414 = property on="moldSelection" class="LstBox (strict)"("Item Names"=w843) -> ()  [unwired: 2 in, 2 out]
          }
          frame Enabled {
          }
        }
        n415 = Enqueue Element(queue=w842, element=T10 {"Message"="Test Edit", "Message Data"=variant}) -> (error out=w841:errorcluster)  [unwired: 2 in, 2 out]
      }
      event "bt_moldInformation": Value Change {
        w864 = enum32{"0", "1", "2", "3", "4", "5"}."0" ("Value (Signaling)")
        # "Enqueue an \"Exit\" message. Note that the Enqueue Element At Opposite End function is used to place this priority \"Exit\" message at the front of the queue ahead of all other messages."
        n416 = event-data() -> ()  [unwired: 1 in, 6 out]
        n417 = property on="Test Button Tab" class="TabCtl (strict)"("Val(Sgnl)"=w864) -> ()  [unwired: 2 in, 2 out]
        n418 = property on="Test Pages Tab" class="TabCtl (strict)"("Val(Sgnl)"=w864) -> ()  [unwired: 2 in, 2 out]
      }
      event "bt_controlParameters": Value Change {
        w866 = enum32{"0", "1", "2", "3", "4", "5"}."1" ("Value (Signaling)")
        # "Enqueue an \"Exit\" message. Note that the Enqueue Element At Opposite End function is used to place this priority \"Exit\" message at the front of the queue ahead of all other messages."
        n419 = event-data() -> ()  [unwired: 1 in, 6 out]
        n420 = property on="Test Button Tab" class="TabCtl (strict)"("Val(Sgnl)"=w866) -> ()  [unwired: 2 in, 2 out]
        n421 = property on="Test Pages Tab" class="TabCtl (strict)"("Val(Sgnl)"=w866) -> ()  [unwired: 2 in, 2 out]
      }
      event "bt_motionProfile": Value Change {
        w868 = enum32{"0", "1", "2", "3", "4", "5"}."2" ("Value (Signaling)")
        # "Enqueue an \"Exit\" message. Note that the Enqueue Element At Opposite End function is used to place this priority \"Exit\" message at the front of the queue ahead of all other messages."
        n422 = event-data() -> ()  [unwired: 1 in, 6 out]
        n423 = property on="Test Button Tab" class="TabCtl (strict)"("Val(Sgnl)"=w868) -> ()  [unwired: 2 in, 2 out]
        n424 = property on="Test Pages Tab" class="TabCtl (strict)"("Val(Sgnl)"=w868) -> ()  [unwired: 2 in, 2 out]
      }
      event "bt_imageUpload": Value Change {
        w874 = enum32{"0", "1", "2", "3", "4", "5"}."3" ("Value (Signaling)")
        # "Enqueue an \"Exit\" message. Note that the Enqueue Element At Opposite End function is used to place this priority \"Exit\" message at the front of the queue ahead of all other messages."
        n425 = event-data() -> ()  [unwired: 1 in, 6 out]
        n426 = call <vilib>:"Application Directory.vi"() -> ("Application Directory"=w871:path)
        n427 = Build Path(base path=w871, name or relative path=path "Data/Image") -> (appended path=w870:path)
        n428 = List Folder(path=w870) -> (filenames=w869:string[])  [unwired: 3 in, 3 out]
        n429 = property on="Image" class="LstBox (strict)"("Item Names"=w869) -> ()  [unwired: 2 in, 2 out]
        n430 = property on="Test Button Tab" class="TabCtl (strict)"("Val(Sgnl)"=w874) -> ()  [unwired: 2 in, 2 out]
        n431 = property on="Test Pages Tab" class="TabCtl (strict)"("Val(Sgnl)"=w874) -> ()  [unwired: 2 in, 2 out]
      }
      event "Add Image": Value Change {
        # "Enqueue an \"Exit\" message. Note that the Enqueue Element At Opposite End function is used to place this priority \"Exit\" message at the front of the queue ahead of all other messages."
        n432 = event-data() -> ()  [unwired: 1 in, 6 out]
        n433 = call <vilib>:"Read PNG File.vi"("path to PNG file"=w877) -> ("image data"=w879:T16, "path"=w876:path)  [unwired: 8 in, 1 out]
        n434 = call <vilib>:"Draw Flattened Pixmap.vi"("image data"=w879) -> ("new picture"=→"image testprm" →"imagework":picture)  [unwired: 8 in]
      }
      event "Image": Value Change {
        # "Enqueue an \"Exit\" message. Note that the Enqueue Element At Opposite End function is used to place this priority \"Exit\" message at the front of the queue ahead of all other messages."
        n435 = event-data() -> ("NewVal"=w888:i32)  [unwired: 1 in, 5 out]
        n436 = property on="Image" class="LstBox (strict)"() -> ("Item Names"=w892:string[])  [unwired: 2 in, 2 out]
        n437 = call <vilib>:"Application Directory.vi"() -> ("Application Directory"=w891:path)
        n438 = Index Array(array=w892, index=w888) -> (element=w883:string)
        n439 = Build Path(base path=w891, name or relative path=path "Data/Image") -> (appended path=w889:path)
        n440 = Build Path(base path=w889, name or relative path=w883) -> (appended path=w881:path)
        n441 = disable-structure shown="Disabled" {
          frame Disabled {
            n442 = Match Pattern(regular expression=".png") -> ()  [unwired: 2 in, 4 out]
            n443 = Match Pattern(regular expression=".jpg") -> ()  [unwired: 2 in, 4 out]
          }
          frame Enabled {
          }
        }
        n444 = String Length(string=w883) -> (length=w887:i32)
        n445 = Subtract(x=w887, y=4) -> (x-y=w885:i32)
        n446 = String Subset(string=w883, offset (0)=w885, length (rest)=4 ("length (rest)")) -> (substring=w882:string)
        n447 = case shown="\".jpg\"" w882 {
          tunnel: w881 -> [w896 w898]
          tunnel: [w894 w897] -> w880
          frame ".jpg" {
            n448 = call <vilib>:"Read JPEG File.vi"("path to JPEG file"=w896) -> ("image data"=w895:T16)  [unwired: 8 in, 2 out]
            n449 = call <vilib>:"Draw Flattened Pixmap.vi"("image data"=w895) -> ("new picture"=w894:picture)  [unwired: 8 in]
          }
          frame ".png", Default {
            n450 = call <vilib>:"Read PNG File.vi"("path to PNG file"=w898) -> ("image data"=w899:T16)  [unwired: 8 in, 2 out]
            n451 = call <vilib>:"Draw Flattened Pixmap.vi"("image data"=w899) -> ("new picture"=w897:picture)  [unwired: 8 in]
          }
        }
        "2D Picture" <- w880
      }
      event "bt_graphLimited": Value Change {
        w903 = enum32{"0", "1", "2", "3", "4", "5"}."4" ("Value (Signaling)")
        # "Enqueue an \"Exit\" message. Note that the Enqueue Element At Opposite End function is used to place this priority \"Exit\" message at the front of the queue ahead of all other messages."
        n452 = event-data() -> ()  [unwired: 1 in, 6 out]
        n453 = property on="Test Button Tab" class="TabCtl (strict)"("Val(Sgnl)"=w903) -> ()  [unwired: 2 in, 2 out]
        n454 = property on="Test Pages Tab" class="TabCtl (strict)"("Val(Sgnl)"=w903) -> ()  [unwired: 2 in, 2 out]
      }
      event "bt_newRecipe": Value Change {
        # "Enqueue an \"Exit\" message. Note that the Enqueue Element At Opposite End function is used to place this priority \"Exit\" message at the front of the queue ahead of all other messages."
        n455 = event-data() -> ()  [unwired: 1 in, 6 out]
        n456 = Enqueue Element(queue=w906, element=T10 {"Message"="New Recipe", "Message Data"=variant}) -> (error out=w905:errorcluster)  [unwired: 2 in, 2 out]
      }
      event "bt_recipeSave": Value Change {
        # "Enqueue an \"Exit\" message. Note that the Enqueue Element At Opposite End function is used to place this priority \"Exit\" message at the front of the queue ahead of all other messages."
        n457 = event-data() -> ()  [unwired: 1 in, 6 out]
        n458 = Enqueue Element(queue=w909, element=T10 {"Message"="Recipe Save", "Message Data"=variant}) -> (error out=w908:errorcluster)  [unwired: 2 in, 2 out]
      }
      event "bt_recipeDelete": Value Change {
        # "Enqueue an \"Exit\" message. Note that the Enqueue Element At Opposite End function is used to place this priority \"Exit\" message at the front of the queue ahead of all other messages."
        n459 = event-data() -> ()  [unwired: 1 in, 6 out]
        n460 = call "Lütfen Şifreyi Giriniz"() -> ("Şifre"=w912:string)  [unwired: 17 in, 2 out]
        n461 = Equal?(x="1234", y=w912) -> (x = y?=w914:bool)
        n462 = case shown="True" w914 {
          tunnel: w911 -> [_ w919]
          tunnel: [_ w917] -> w910
          frame False {
            n463 = One Button Dialog(message="Şifre Yanlış!", button name ("OK")="TAMAM") -> ()  [unwired: 1 out]
          }
          frame True {
            n464 = Enqueue Element(queue=w919, element=T10 {"Message"="Recipe Delete", "Message Data"=variant}) -> (error out=w917:errorcluster)  [unwired: 2 in, 2 out]
          }
        }
      }
      event "bt_recipeSend": Value Change {
        # "Enqueue an \"Exit\" message. Note that the Enqueue Element At Opposite End function is used to place this priority \"Exit\" message at the front of the queue ahead of all other messages."
        n465 = event-data() -> ()  [unwired: 1 in, 1 out]
        n466 = Enqueue Element(queue=w922, element=T10 {"Message"="Recipe Send", "Message Data"=variant}) -> (error out=w921:errorcluster)  [unwired: 2 in, 2 out]
      }
      event "moldSelection": Value Change {
        # "Enqueue an \"Exit\" message. Note that the Enqueue Element At Opposite End function is used to place this priority \"Exit\" message at the front of the queue ahead of all other messages."
        n467 = event-data() -> ()  [unwired: 1 in, 6 out]
        n468 = flat-sequence {
          tunnel: w923 -> [w963]
          frame #0 {
            n469 = Index Array(array=w963, index=3) -> (element=w966:string)
            n470 = Unflatten From XML(xml string=w966, type="" ("anything")) -> (value=w962:string)  [unwired: 1 in, 1 out]
            n471 = call <vilib>:"Application Directory.vi"() -> ("Application Directory"=w961:path)
            n472 = Build Path(base path=w961, name or relative path=path "Data/Image") -> (appended path=w969:path)
            n473 = List Folder(path=w969) -> (filenames=w970:string[])  [unwired: 3 in, 3 out]
            n474 = Search 1D Array(1D array=w970, element=w962) -> (index of element=w972:i32)  [unwired: 1 in]
            n475 = Greater Or Equal To 0?(x=w972) -> (x >= 0?=w971:bool)
            n476 = Select(t=w972, s=w971, f=nan) -> (s? t:f=w974:dbl)
            n477 = Build Path(base path=w969, name or relative path=w962) -> (appended path=w968:path)
            n478 = property on="Image" class="LstBox (strict)"("Value"=w974) -> ()  [unwired: 2 in, 2 out]
            n479 = call <vilib>:"Read PNG File.vi"("path to PNG file"=w968) -> ("image data"=w960:T16)  [unwired: 8 in, 2 out]
            n480 = call <vilib>:"Draw Flattened Pixmap.vi"("image data"=w960) -> ("new picture"=w959:picture)  [unwired: 8 in]
            n481 = property on="2D Picture" class="Pict"("Value"=w959) -> ()  [unwired: 2 in, 2 out]
          }
          frame #1 {
          }
        }
        n482 = property on="moldSelection" class="LstBox (strict)"() -> ("Item Names"=w930:string[], "Value"=w945:i32)  [unwired: 2 in, 2 out]
        n483 = call <vilib>:"Application Directory.vi"() -> ("Application Directory"=w944:path)
        n484 = Index Array(array=w930, index=w945) -> (element=w928:string)
        n485 = Build Path(base path=w944, name or relative path=path "Data/Receipt") -> (appended path=w950:path)
        n486 = Concatenate Strings(w928, ".xml") -> (w949:string)
        n487 = List Folder(path=w950) -> (filenames=w946:string[])  [unwired: 3 in, 3 out]
        n488 = Equal?(x=w928, y="") -> (x = y?=w927:bool)
        n489 = Select(t=T15."Disabled and Grayed Out" ("Disabled"), s=w927, f=T15."Enabled" ("Disabled")) -> (s? t:f=w926:T15)
        n490 = Search 1D Array(1D array=w946, element=w949) -> (index of element=w947:i32)  [unwired: 1 in]
        n491 = Greater Or Equal To 0?(x=w947) -> (x >= 0?=w948:bool)
        n492 = property on="bt_recipeSend" class="Bool"("DisabledEnum"=w926) -> ()  [unwired: 2 in, 2 out]
        n493 = Select(t=w949, s=w948, f="") -> (s? t:f=w952:string)
        n494 = Build Path(base path=w950, name or relative path=w952) -> (appended path=w951:path)
        n495 = call-poly <vilib>:"Read From XML File.vi"("XML File Path"=w951) -> ("XML Elements"=w923:string[])  [unwired: 8 in, 2 out]
        n496 = Index Array(array=w923, index=0) -> (element=w954:string)
        n497 = Index Array(array=w923, index=1) -> (element=w933:string)
        n498 = Index Array(array=w923, index=2) -> (element=w953:string)
        n499 = Unflatten From XML(xml string=w953, type=T4 {"TDC"=0.0, "S1"=0.0, "P1"=0.0, "S2"=0.0, "BDC"=0.0, "S3"=0.0, "Bekleme Süresi"=0.0} ("HAREKET PROFİLİ")) -> (value=w958:T4)  [unwired: 1 in, 1 out]
        n500 = Unflatten From XML(xml string=w954, type=T12 {"Parça No"="111445", "Seri No"="565", "Müşteri"="Mercedes-Benz", "Kalıp No"="6666", "Kuvvet Limiti [kN]"="1000", "Kuvvet Limiti [kN] 2"="1000"} ("KALIP BİLGİLERİ")) -> (value=w957:T12)  [unwired: 1 in, 1 out]
        n501 = Unflatten From XML(xml string=w933, type=T3 {"Kuvvet Limit"="", "Grafik Limit"=""} ("anything")) -> (value=w931:T3)  [unwired: 1 in, 1 out]
        n502 = property on="HAREKET PROFİLİ" class="Clust (strict)"("Value"=w958) -> ()  [unwired: 2 in, 2 out]
        n503 = property on="KALIP BİLGİLERİ" class="Clust (strict)"("Value"=w957) -> ()  [unwired: 2 in, 2 out]
        n504 = Unbundle By Name(w957) -> ("Parça No"=w955:string, "Seri No"=w956:string)
        n505 = property on="KONTROL PARAM" class="Clust (strict)"("Value"=w931) -> ()  [unwired: 2 in, 2 out]
        n506 = local write "pieceNo"(w955) -> ()
        n507 = local write "serialNo"(w956) -> ()
        n508 = property on="Mold Choice Tab" class="TabCtl (strict)"("Val(Sgnl)"=enum32{"0", "1", "2"}."1" ("Value (Signaling)")) -> ()  [unwired: 2 in, 2 out]
      }
      event "addReferance": Value Change {
        # "Enqueue an \"Exit\" message. Note that the Enqueue Element At Opposite End function is used to place this priority \"Exit\" message at the front of the queue ahead of all other messages."
        n509 = event-data() -> ()  [unwired: 1 in, 1 out]
        n510 = Enqueue Element(queue=w976, element=T10 {"Message"="Add Referance", "Message Data"=variant}) -> (error out=w975:errorcluster)  [unwired: 2 in, 2 out]
      }
      event "deleteReferance": Value Change {
        # "Enqueue an \"Exit\" message. Note that the Enqueue Element At Opposite End function is used to place this priority \"Exit\" message at the front of the queue ahead of all other messages."
        n511 = event-data() -> ()  [unwired: 1 in, 1 out]
        n512 = Enqueue Element(queue=w979, element=T10 {"Message"="Delete Reference", "Message Data"=variant}) -> (error out=w978:errorcluster)  [unwired: 2 in, 2 out]
      }
    }
    n513 = call "Error Handler - Event Handling Loop.vi"("error in (no error)"=w764, "Message Queue"=w766) -> ("dup error in"=w765:errorcluster)  [unwired: 8 in, 1 out]
  }
  n514 = Merge Errors(w17, w18) -> (w13:errorcluster)
  n515 = call <vilib>:"Simple Error Handler.vi"("error in (no error)"=w13) -> ()  [unwired: 4 in, 5 out]
  n516 = disable-structure shown="Disabled" {
    frame Disabled {
      (unwired) T4 {"TDC"=0.0, "S1"=0.0, "P1"=0.0, "S2"=0.0, "BDC"=0.0, "S3"=0.0, "Bekleme Süresi"=0.0} ("HAREKET PROFİLİ")
      (unwired) T17 {"Parça No"="111445", "Seri No"="565", "Müşteri"="Mercedes-Benz", "Kalıp No"="6666", "Kuvvet Limiti [kN]"="1000"} ("KALIP BİLGİLERİ")
      n517 = Unflatten From XML() -> ()  [unwired: 3 in, 2 out]
      n518 = property on="Image" class="LstBox (strict)" props=["Item Names"]() -> ()  [unwired: 3 in, 2 out]
      n519 = Unflatten From XML() -> ()  [unwired: 3 in, 2 out]
    }
    frame Enabled {
    }
  }
